vi "Dashboard Main.vi"() -> ()   [LabVIEW 2019]
uses:
  <vilib>/Utility/miscctls.llb/LVRowAndColumnTypeDef.ctl
  <vilib>/event_ctls.llb/eventvkey.ctl
  <vilib>/Rock Robotics/Network Tables/NT Write Boolean.vi
  <vilib>/Rock Robotics/WPI/Dashboard/WPI_DashboardLogging Global.vi
  <vilib>/Utility/file.llb/Write Delimited Spreadsheet (string).vi
panel:
  in  "Camera Settings Right":T1={"Frame Rate"=30, "Compression"=30, "Size"=1, "DB Camera Config"=FALSE} {"Frame Rate" scale=1.0..30.0; "Compression" scale=100.0..-1.0; "Size" items=["640x480", "320x240", "160x120"]}
  in  "Camera Name Right":string(combo)="No Camera Selection"
  out "Camera Perf":string
  in  "Camera Settings":T1={"Frame Rate"=30, "Compression"=30, "Size"=1, "DB Camera Config"=FALSE} {"Frame Rate" scale=1.0..30.0; "Compression" scale=100.0..-1.0; "Size" items=["640x480", "320x240", "160x120"]}
  in  "TCP":refnum<k5>
  in  "Rec Mode":enum32{"Stop", "Record", "Playback"}(radio)
  out "Robot IP":string
  out "Image Message":string="Timeout in Camera Communications"
  in  "Dashboard Tab":T2(tab)
  in  "Select Auto":string(combo)="Select Autonomous ..."
  out "NT Connection":bool
  out "JS1 Z":dbl(slide) scale=-1.0..1.0 scale format="%#_2e"
  out "JS1 Graph":cluster{"X":dbl, "Y":dbl}[](graph)
  out "JS1 Buttons":T3
  out "JS2 Z":dbl(slide) scale=-1.0..1.0 scale format="%#_2e"
  out "JS2 Graph":cluster{"X":dbl, "Y":dbl}[](graph)
  out "JS2 Buttons":T3
  out "Mode":T4(ring)=enum."Auto Disabled"
  out "Right Camera Perf":cluster{"Bandwidth (Mbps)":dbl, "FPS":dbl}
  out "Camera Image Right":T5(plugin-control)
  in  "DB/String 9":string
  in  "DB/String 8":string
  in  "DB/String 7":string
  in  "DB/String 6":string
  in  "DB/String 5":string
  in  "DB/String 4":string
  in  "DB/String 3":string
  in  "DB/String 2":string
  in  "DB/String 1":string
  in  "DB/String 0":string
  in  "DB/Slider 0":dbl(slide) scale=0.0..5.0
  in  "DB/Slider 1":dbl(slide) scale=0.0..5.0
  in  "DB/Slider 2":dbl(slide) scale=0.0..5.0
  in  "DB/Slider 3":dbl(slide) scale=0.0..5.0
  out "DB/LED 3":bool
  out "DB/LED 2":bool
  out "DB/LED 1":bool
  out "DB/LED 0":bool
  in  "DB/Button 3":bool
  in  "DB/Button 2":bool
  in  "DB/Button 1":bool
  in  "DB/Button 0":bool caption="New Name"
  in  "Test Slider":dbl(slide) scale=0.0..100.0 scale format="%#_3g"
  in  "On/Off":bool caption="Solenoid"
  in  "Test Name":u16(ring) items=["Select the test to run..."]
  in  "Test Tree":string(tree)
  in  "Motor":cluster{"Value":dbl, "Enable":bool} {"Value" scale=-1.0..1.0 scale format="%#_3g"}
  out "Progress":T6 {"Test Progress" scale=0.0..100.0}
  in  "Rev/Fwd":cluster{"Forward":bool, "Reverse":bool}
  in  "Test Ring":u16(ring) items=["Monochrome", "Color"]
  out "Cmd Status":string
  in  "Execute Command":bool
  in  "Command Params":string[][](table)
  in  "Command Selection":i32(listbox)
  in  "CheckList":i32(listbox)
  out "Tree":string(tree)
  out "Drive":enum32{"Controls", "Indicators"}(tab)
  in  "Left Low Gear P":dbl
  in  "Left Low Gear I":dbl
  in  "Left Low Gear D":dbl
  in  "Left Low Gear F":dbl
  in  "Left High Gear P":dbl
  in  "Left High Gear I":dbl
  in  "Left High Gear D":dbl
  in  "Left High Gear F":dbl
  in  "Right Low Gear P":dbl
  in  "Right Low Gear I":dbl
  in  "Right Low Gear D":dbl
  in  "Right Low Gear F":dbl
  in  "Right High Gear P":dbl
  in  "Right High Gear I":dbl
  in  "Right High Gear D":dbl
  in  "Right High Gear F":dbl
  out "Current Left High Gear F":dbl
  out "Current Left High Gear D":dbl
  out "Current Left High Gear P":dbl
  out "Current Left High Gear I":dbl
  out "Current Right High Gear F":dbl
  out "Current Right High Gear D":dbl
  out "Current Right High Gear P":dbl
  out "Current Right High Gear I":dbl
  out "Current Right Low Gear F":dbl
  out "Current Right Low Gear D":dbl
  out "Current Right Low Gear I":dbl
  out "Current Right Low Gear P":dbl
  out "Current Left Low Gear F":dbl
  out "Current Left Low Gear D":dbl
  out "Current Left Low Gear I":dbl
  out "Current Left Low Gear P":dbl
  out "Auto Targeting":enum32{"Controls", "Indicators"}(tab)
  in  "AutoTarget D":dbl
  in  "AutoTarget I":dbl
  in  "AutoTarget P":dbl
  out "Current AutoTarget D":dbl
  out "Current AutoTarget I":dbl
  out "Current AutoTarget P":dbl
  out "Cardinal Points":enum32{"Controls", "Indicators"}(tab)
  in  "Turret West":dbl
  in  "Turret South":dbl
  in  "Turret Safety":dbl
  in  "Turret North":dbl
  in  "Turret East":dbl
  out "Current Turret Safety":dbl
  out "Current Turret West":dbl
  out "Current Turret South":dbl
  out "Current Turret East":dbl
  out "Current Turret North":dbl
  out "Climb":enum32{"Controls", "Indicators"}(tab)
  in  "Climb I":dbl
  in  "Climb P":dbl
  in  "Climb D":dbl
  out "Current Climb D":dbl
  out "Current Climb I":dbl
  out "Current Climb P":dbl
  out "Intake":enum32{"Controls", "Indicators"}(tab)
  in  "Intake Speed":dbl
  in  "Magazine Speed":dbl
  out "Current Intake Speed":dbl
  out "Current Magazine Speed":dbl
  out "Match Color":string
  in  "Auto play selection":string
  out "Camera Image":T5(plugin-control)
  out "Background":bool
  in  "Camera Name":string(combo)="No Camera Selection"
  # "HW"
  # "HW"
  # "Joysticks"
  # "Drive Motors"
  # "Front"
  # "Right"
  # "Left"
  # "Back"
  # "This tab is a great place for autonomous settings and robot-specific values.\nPlace controls and indicators inside this tab and match name to\nDashboard Variables on robot. You can also delete this comment."
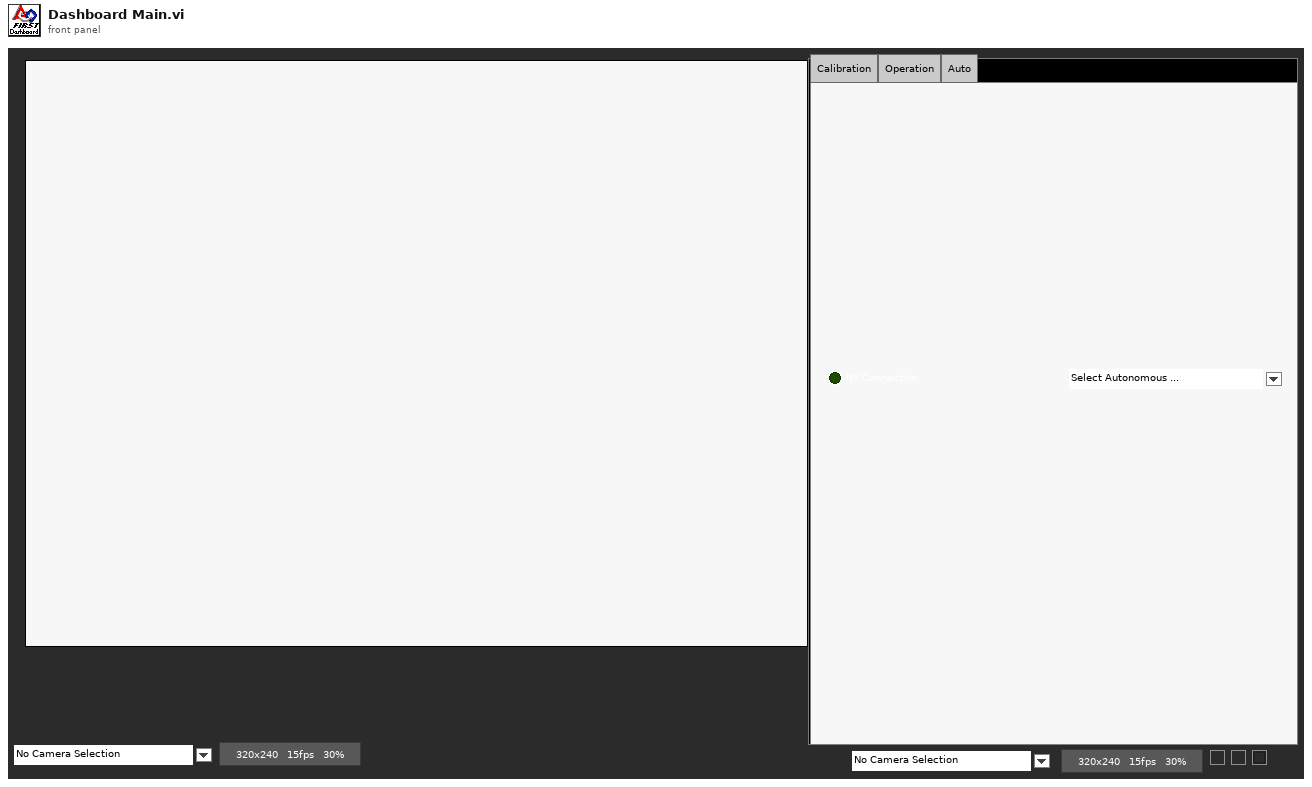
[diagram p1: front panel]
types:
  T1 = cluster{"Frame Rate":i32, "Compression":i32, "Size":u16, "DB Camera Config":bool}
  T2 = enum32{"Drive", "Camera", "Basic", "Custom", "Test", "Commands", "Checklist", "Variables", "Calibration", "Operation", "Auto"}
  T3 = cluster{bool, bool, bool, bool, bool, bool, bool, bool, bool, bool, bool, bool}
  T4 = enum8{"Tele-Op Disabled", "Tele-Op Enabled", "Auto Disabled", "Auto Enabled", "Test Disabled", "Test Enabled", "Disconnected", "No Code", "E-Stop"}
  T5 = typedef "IMAQ Image.ctl" = refnum<image>
  T6 = cluster{"Test Progress":u8, "Test Progress Text":string}
  T7 = enum16{"open", "replace", "create", "open or create", "replace or create", "replace or create with confirmation"}
  T8 = cluster{"Save Path":path, "Interval (s)":dbl, "Keep":i32}
  T9 = enum32{"Drive", "Camera", "Basic", "Custom", "Test", "Commands", "Checklist", "Variables"}
  T10 = typedef "Image Type" = u32
  T11 = cluster{"IDs":cluster{"RPC field ID":u16, "Unique ID":u16}, "String":string}
  T12 = cluster{"Error Strings":string, "Disable Counts":cluster{u16, u16}, "Rail Faults":cluster{u16, u16, u16}, "Robot IP":string, "DB Mode":u8, "Event Info":cluster{"Name":string, "Type":u8, "Number":u16, "Replay":u8}}
  T13 = cluster{"Storage":cluster{"Disk Free":u64, "RAM Block":u32, "RAM free":u32}, "CPU Utilization":cluster{"CPU % ISR":sgl, "CPU % Time Crit":sgl, "CPU % Timed Str":sgl, "CPU % High":sgl, "CPU % Above":sgl, "CPU % Normal":sgl, "CPU % Low":sgl}, "CAN":cluster{"% Bus Utilization":sgl, "Bus Off Cnt":u32, "TX_FIFO Full Cnt":u32, "Receive Error Cnt":u8, "Transmit Error Cnt":u8}, "HID":cluster{"HID Outputs":u32, "Rumble Low":u16, "Rumble High":u16}[]}
  T14 = cluster{"Status bits":cluster{"Test Mode":bool, "Autonomous":bool, "Enabled":bool, "Code Start":bool, "Brownout":bool, "Reserved 2":bool, "Reserved 3":bool, "E-Stop":bool}, "Code Trace":cluster{"Disabled":bool, "TeleOp":bool, "Auto":bool, "Test":bool}, "Controller Type":enum16{"unknown", "cRIO", "roboRio"}, "Code?":enum16{"unknown", "noCode", "code"}, "Battery V":dbl}
  T15 = cluster{"Control Bits":cluster{"TestMode":bool, "Autonomous":bool, "Enabled":bool, "FMS Present":bool, bool, bool, bool, "E-Stop":bool}, "Team Station ":u8, "Countdown":sgl, "Joystick Values":cluster{"Axes":dbl[], "Buttons":bool[], "POVs":i16[]}[]}
  T16 = cluster{"Axes":dbl[], "Buttons":bool[], "POVs":i16[]}[]
  T17 = cluster{"Axes":dbl[], "Buttons":bool[], "POVs":i16[]}
  T18 = cluster{"Buttons[0]":bool, "Buttons[1]":bool, "Buttons[2]":bool, "Buttons[3]":bool, "Buttons[4]":bool, "Buttons[5]":bool, "Buttons[6]":bool, "Buttons[7]":bool, "Buttons[8]":bool, "Buttons[9]":bool, "Buttons[10]":bool, "Buttons[11]":bool}
  T19 = cluster{"Camera Image":refnum<vi>, "Dashboard Tab":refnum<vi>, "Background":refnum<vi>, "Rec Mode":refnum<vi>, "Test Slider":refnum<vi>, "On/Off ":refnum<vi>, "Test Ring":refnum<vi>, "Rev/Fwd":refnum<vi>, "Test Name":refnum<vi>, "Motor":refnum<vi>, "Progress":refnum<vi>, "CheckList":refnum<vi>, "Tree":refnum<vi>, "Test Tree":refnum<vi>, "Command Params":refnum<vi>, "Command Selection":refnum<vi>, "Execute Command":refnum<vi>, "Cmd Status":refnum<vi>, "Camera Settings":refnum<vi>, "Camera Name":refnum<vi>, "Camera Perf":refnum<vi>, "Camera Settings Right":refnum<vi>, "Camera Name Right":refnum<vi>, "Camera Image Right":refnum<vi>}
  T20 = cluster{"Global Rectangle":i32[], "Contours":cluster{"Contour Type":u32, "ROI Type":u32, "Points":i32[]}[]}
  T21 = cluster{"Camera Name":string, string, "Saved DB Images Info":cluster{"Save Path":path, "Interval (s)":dbl, "Keep":i32}}
  T22 = cluster{"Camera Name Right":string, string, "Saved DB Images Info":cluster{"Save Path":path, "Interval (s)":dbl, "Keep":i32}}
  T23 = cluster{"Operation":enum16{"Update", "Clear"}, "Color Box":u32}[]
  T24 = typedef "eventvkey.ctl" = enum16{"ASCII", "Enter", "Return", "Shift", "Ctrl", "Alt", "Cmd", "Opt", "Caps", "NumLock", "Clear", "Break", "Up", "Down", "Left", "Right", "Insert", "Delete", "Home", "End", "PageUp", "PageDown", "Escape", "Help", "Pause", "ScrollLock", "F1", "F2", "F3", "F4", "F5", "F6", "F7", "F8", "F9", "F10", "F11", "F12", "F13", "F14", "F15", "F16", "F17", "F18", "F19", "F20", "F21", "F22", "F23", "F24", "Play", "VolumeUp", "VolumeDown", "Mute", "Two Byte Char"}
  T25 = cluster{"Image Size":bool, "Image Type":bool, "Pixel Value":bool, "ROI Information":bool, "Zoom Factor":bool}
  T26 = cluster{"Operation":enum16{"Update", "Clear"}, "Color Box":u32}
  T27 = typedef "LVRowAndColumnTypeDef.ctl" = cluster{"Row":i32, "Column":i32}
  T28 = cluster{"Shift":bool, "Ctrl":bool, "Alt":bool, "Cmd":bool, "Opt":bool}
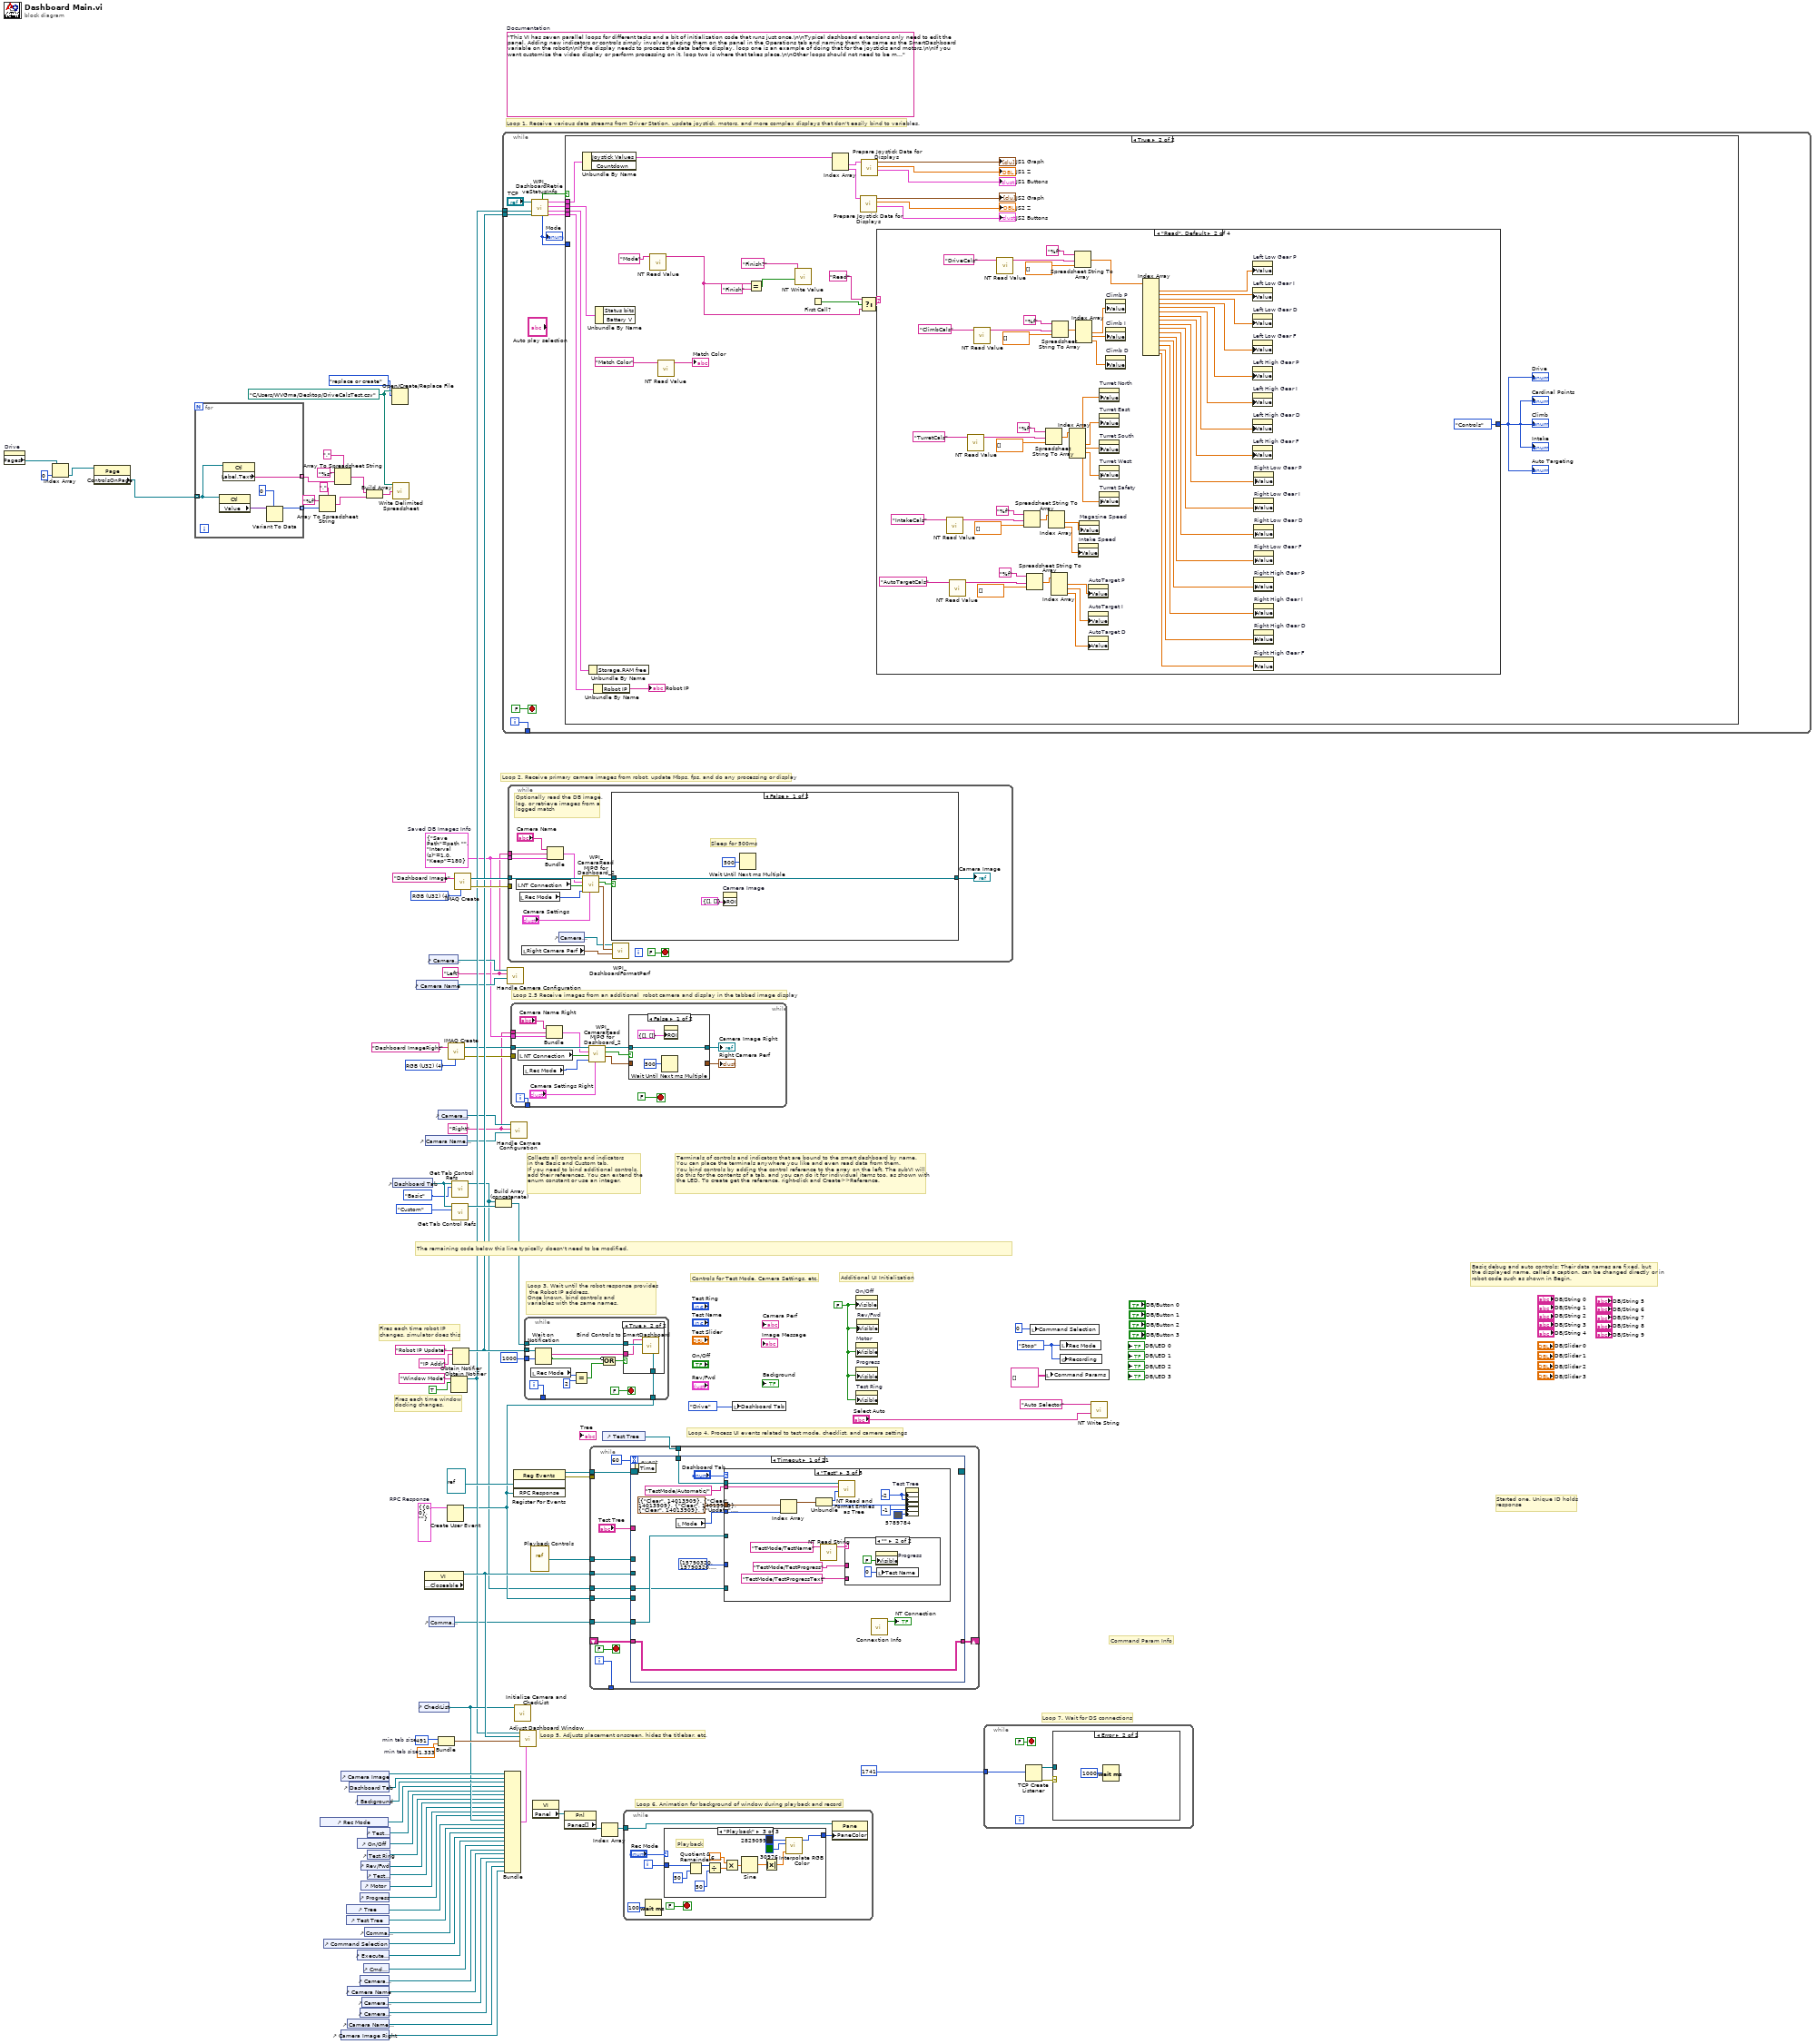
[diagram p0: block diagram]
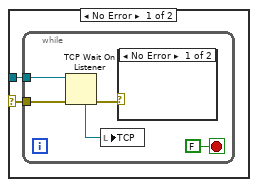
[diagram p3: hidden frame]
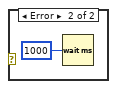
[diagram p4: hidden frame]
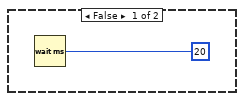
[diagram p5: hidden frame]
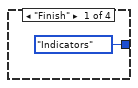
[diagram p6: hidden frame]
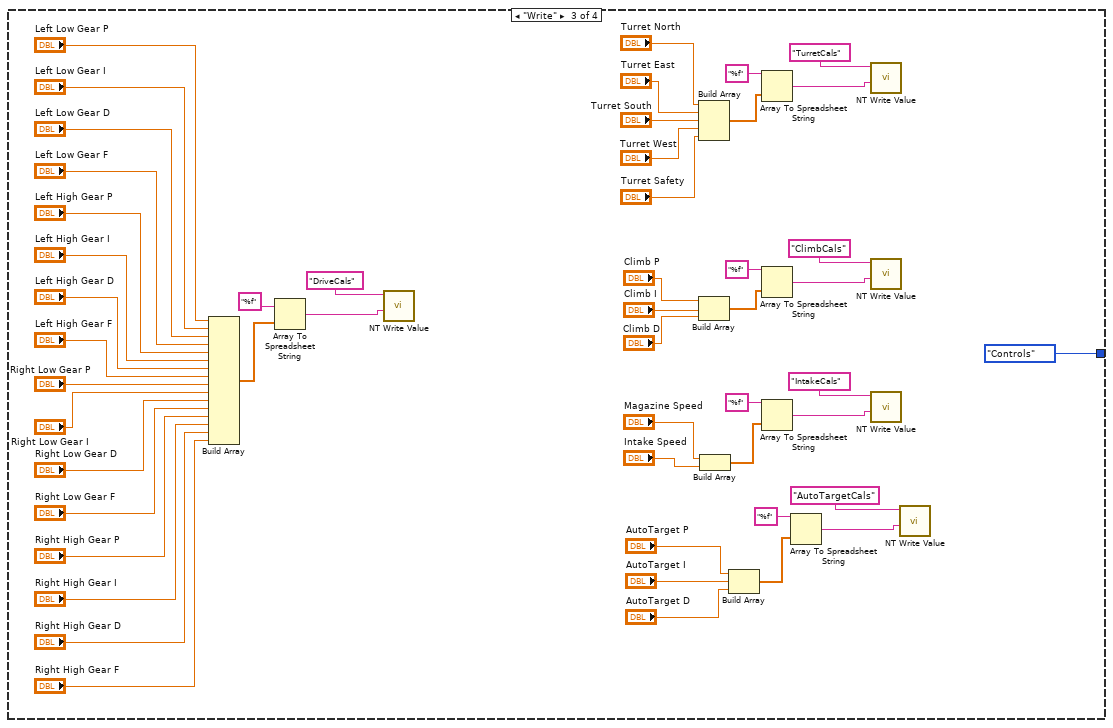
[diagram p7: hidden frame]
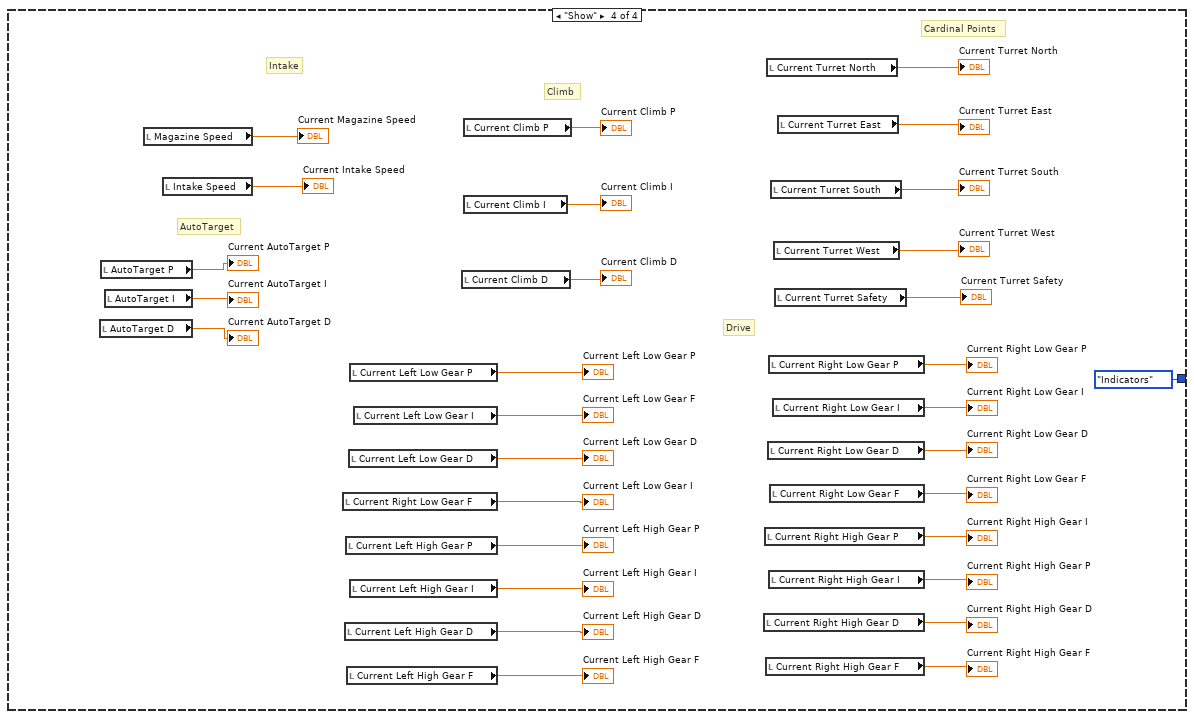
[diagram p8: hidden frame]
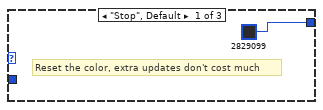
[diagram p9: hidden frame]
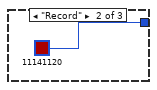
[diagram p10: hidden frame]
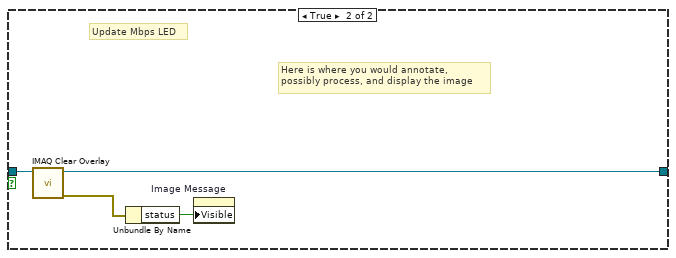
[diagram p12: hidden frame]
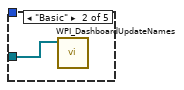
[diagram p14: hidden frame]
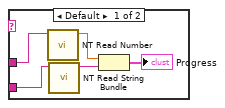
[diagram p15: hidden frame]
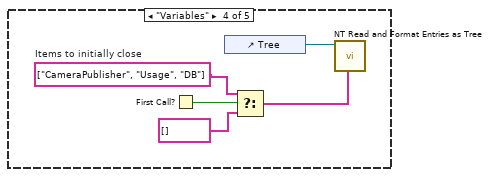
[diagram p16: hidden frame]
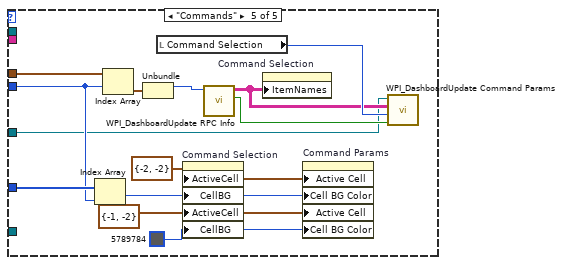
[diagram p17: hidden frame]
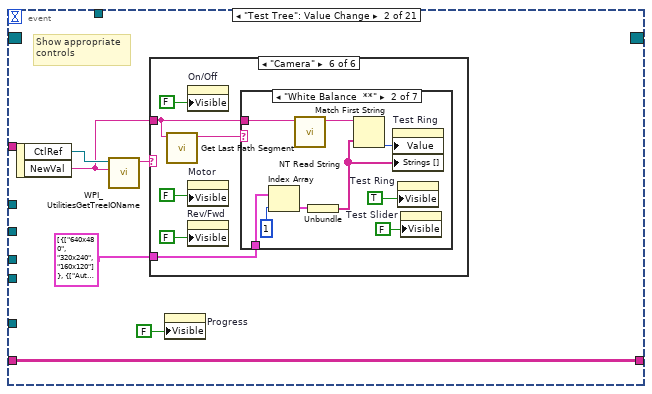
[diagram p18: hidden frame]
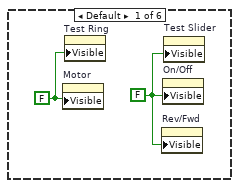
[diagram p19: hidden frame]
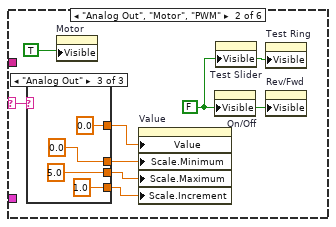
[diagram p20: hidden frame]
diagram:
  w2 = path "C:/Users/WVGma/Desktop/DriveCalsTest.csv" ("file path (dialog if empty)")
  w18 = T8 {"Save Path"=path "", "Interval (s)"=1.0, "Keep"=180}  # Saved DB Images Info
  w17 = "Right"
  w16 = "Left"
  w28 = T10 4 items=["Grayscale (U8)", "Grayscale (I16)", "Grayscale (SGL)", "Complex (CSG)", "RGB (U32)", "HSL (U32)", "RGB (U64)"] ("Image Type")
  w44 = T11 {"IDs"={"RPC field ID"=0, "Unique ID"=0}, "String"=""}  # RPC Response
  w67 = 491  # min tab size
  w66 = 1.333  # min tab size
  w74 = enum32{"Stop", "Record", "Playback"}."Stop" ("Rec Mode")
  w51 = FALSE ("Visible")
  (unwired) "This VI has seven parallel loops for different tasks and a bit of initialization code that runs just once.\n\nTypical dashboard extensions only need to edit the panel. Adding new indicators or controls simply involves placing them on the panel in the Operations tab and naming them the same as the SmartDashboard variable on the robot\n\nIf the display needs to process the data before display, loop one is an example of doing that for the joysticks and motors.\n\nIf you want customize the video display or perform processing on it, loop two is where that takes place.\n\nOther loops should not need to be modified. They are pretty standard, and document the task they perform."  # Documentation
  w91 = T10 4 items=["Grayscale (U8)", "Grayscale (I16)", "Grayscale (SGL)", "Complex (CSG)", "RGB (U32)", "HSL (U32)", "RGB (U64)"] ("Image Type")
  # "Loop 2.5 Receive images from an additional  robot camera and display in the tabbed image display"
  # "Command Param Info"
  # "Started one, Unique ID holds\nresponse"
  # "Loop 7. Wait for DS connections"
  # "Basic debug and auto controls: Their data names are fixed, but\nthe displayed name, called a caption, can be changed directly or in\nrobot code such as shown in Begin."
  # "Controls for Test Mode, Camera Settings, etc."
  # "Additional UI Initialization"
  # "Loop 6. Animation for background of window during playback and record"
  # "Fires each time robot IP\nchanges, simulator does this"
  # "Fires each time window\ndocking changes."
  # "Collects all controls and indicators\nin the Basic and Custom tab.\nIf you need to bind additional controls,\nadd their references. You can extend the\nenum constant or use an integer."
  # "The remaining code below this line typically doesn't need to be modified."
  # "Loop 4. Process UI events related to test mode, checklist, and camera settings"
  # "Terminals of controls and indicators that are bound to the smart dashboard by name.\nYou can place the terminals anywhere you like and even read data from them.\nYou bind controls by adding the control reference to the array on the left. The subVI will\ndo this for the contents of a tab, and you can do it for individual items too, as shown with\nthe LED. To create get the reference, right-click and Create>>Reference."
  # "Loop 3. Wait until the robot response provides\n the Robot IP address.\nOnce known, bind controls and\nvariables with the same names."
  # "Loop 5. Adjusts placement onscreen, hides the titlebar, etc."
  # "Loop 1. Receive various data streams from Driver Station, update joystick, motors, and more complex displays that don't easily bind to variables."
  # "Loop 2. Receive primary camera images from robot, update Mbps, fps, and do any processing or display"
  n1 = property on="Drive" class="TabCtl (strict)"() -> ("Pages"=w13:refnum<vi>[])  [unwired: 2 in, 2 out]
  n2 = Index Array(array=w13, index=0) -> (element=w14:refnum<vi>)
  n3 = property class="Page"(reference=w14) -> ("ControlsOnPage"=w15:refnum<vi>[])  [unwired: 1 in, 2 out]
  n4 = for {
    tunnel: w15 -> [w95] mode=indexing
    tunnel: [w96] -> w11 mode=indexing
    tunnel: [w92] -> w8 mode=indexing
    n5 = property class="Ctl"(reference=w95) -> ("Value"=w94:variant)  [unwired: 1 in, 2 out]
    n6 = property class="Ctl"(reference=w95) -> ("Label.Text"=w96:string)  [unwired: 1 in, 2 out]
    n7 = Variant To Data(type=0, Variant=w94) -> (data=w92:i32)  [unwired: 1 in, 1 out]
  }
  n8 = Array To Spreadsheet String(delimiter (Tab)=",", array=w8, 3:"%f" ("format string")) -> (spreadsheet string=w4:string)
  n9 = control-ref of="Rec Mode"() -> (w57:refnum<vi>)
  n10 = control-ref of="Command Selection"() -> (w43:refnum<vi>)
  n11 = Array To Spreadsheet String(delimiter (Tab)=",", array=w11, 3:"%s" ("format string")) -> (spreadsheet string=w5:string)
  n12 = control-ref of="Camera Image Right"() -> (w21:refnum<vi>)
  n13 = control-ref of="Camera Image"() -> (w69:refnum<vi>)
  n14 = control-ref of="Tree"() -> (w61:refnum<vi>)
  n15 = control-ref of="Test Tree"() -> (w60:refnum<vi>)
  n16 = control-ref of="Camera Name"() -> (w34:refnum<vi>)
  n17 = control-ref of="Camera Name Right"() -> (w22:refnum<vi>)
  n18 = control-ref of="Dashboard Tab"() -> (w68:refnum<vi>)
  n19 = control-ref of="Execute Command"() -> (w45:refnum<vi>)
  n20 = control-ref of="Background"() -> (w64:refnum<vi>)
  n21 = control-ref of="On/Off"() -> (w55:refnum<vi>)
  n22 = control-ref of="Progress"() -> (w52:refnum<vi>)
  n23 = control-ref of="Camera Settings"() -> (w35:refnum<vi>)
  n24 = control-ref of="Camera Settings Right"() -> (w23:refnum<vi>)
  n25 = control-ref of="Rev/Fwd"() -> (w53:refnum<vi>)
  n26 = control-ref of="Motor"() -> (w58:refnum<vi>)
  n27 = control-ref of="Camera Perf"() -> (w33:refnum<vi>)
  n28 = control-ref of="Cmd Status"() -> (w39:refnum<vi>)
  n29 = control-ref of="Command Params"() -> (w46:refnum<vi>)
  n30 = Build Array(w5, w4) -> (w3:string[])
  n31 = control-ref of="Test Slider"() -> (w56:refnum<vi>)
  n32 = control-ref of="Test Ring"() -> (w54:refnum<vi>)
  n33 = control-ref of="Test Name"() -> (w59:refnum<vi>)
  n34 = Open/Create/Replace File(file path (use dialog)=w2, operation (0:open)=T7."replace or create") -> ()  [unwired: 4 in, 3 out]
  n35 = call-poly <vilib>:"Write Delimited Spreadsheet.vi"("file path (dialog if empty)"=w2, "1D data"=w3) -> ()  [unwired: 12 in, 2 out]
  n36 = control-ref of="Dashboard Tab"() -> (w72:refnum<vi>)
  n37 = control-ref of="Camera Name"() -> (w36:refnum<vi>)
  n38 = control-ref of="CheckList"() -> (w62:refnum<vi>)
  n39 = property class="VI" props=["Front Panel.Closeable"]() -> (reference out=w73:refnum<vi>)  [unwired: 2 in, 2 out]
  n40 = control-ref of="Camera Name Right"() -> (w24:refnum<vi>)
  n41 = control-ref of="Camera Settings"() -> (w37:refnum<vi>)
  n42 = control-ref of="Command Params"() -> (w38:refnum<vi>)
  n43 = control-ref of="Camera Settings Right"() -> (w25:refnum<vi>)
  n44 = Bundle("min tab size"=w67, "min tab size"=w66) -> (w65:cluster{"min tab size":i32, "min tab size":dbl})  [unwired: 1 in]
  n45 = Create User Event(user event datatype=w44) -> (user event=w40:refnum<user-event>)  [unwired: 1 in, 1 out]
  n46 = call "IMAQ Create"("Image Name"="Dashboard ImageRight", "Image Type"=w28) -> ("New Image"=w27:T5, "error out"=w26:errorcluster)  [unwired: 2 in, 1 out]
  n47 = Obtain Notifier(name (unnamed)="Window Mode", notification data type=TRUE) -> (notifier out=w49:refnum<notifier>)  [unwired: 2 in, 2 out]
  n48 = call <vilib>:"Get Tab Control Refs.vi"("Page Index"=T9."Basic" ("Dashboard Tab"), "TabControl in"=w72) -> ("ControlsOnPage"=w32:refnum<vi>[])  [unwired: 9 in]
  n49 = call <vilib>:"Get Tab Control Refs.vi"("Page Index"=T9."Custom" ("Dashboard Tab"), "TabControl in"=w72) -> ("ControlsOnPage"=w71:refnum<vi>[])  [unwired: 9 in]
  n50 = Obtain Notifier(name (unnamed)="Robot IP Update", notification data type="IP Addr" ("name (unnamed)")) -> (notifier out=w50:refnum<notifier>)  [unwired: 2 in, 2 out]
  n51 = call "IMAQ Create"("Image Name"="Dashboard Image", "Image Type"=w91) -> ("New Image"=w89:T5, "error out"=w88:errorcluster)  [unwired: 2 in, 1 out]
  n52 = Build Array (concatenate)(w32, w71) -> (w70:refnum<vi>[])
  n53 = while {
    tunnel: [w106] -> _
    tunnel: w50 -> [w100]
    tunnel: w49 -> [w97]
    i -> [w106]
    stop <- FALSE stop-if-true
    n54 = call <vilib>:"WPI_DashboardRetrieveStatusInfo.vi"("Binding Refnum"=w100, "Window Mode Notifier"=w97, "TCP Cnx"="TCP") -> ("Power and Errors"=w101:T12, "Robot Metrics"=w104:T13, "Status Info"=w105:T14, "Control Info"=w102:T15, "Robot Mode"=w99:T4, "Process?"=w103:bool)  [unwired: 3 in]
    "Mode" <- w99
    n55 = case shown="True" w103 {
      tunnel: w105 -> [_ w133]
      tunnel: w104 -> [_ w132]
      tunnel: w102 -> [_ w131]
      tunnel: w101 -> [_ w130]
      tunnel: w99 -> [_ _]
      frame False {
        n56 = Wait (ms)(milliseconds to wait=u32 20) -> ()  [unwired: 1 out]
      }
      frame True {
        n57 = Unbundle By Name(w131) -> ("Joystick Values"=w129:T16)  [unwired: 1 out]
        n58 = Unbundle By Name(w132) -> ()  [unwired: 1 out]
        n59 = Unbundle By Name(w130) -> ("Robot IP"=→"Robot IP":string)
        n60 = Unbundle By Name(w133) -> ()  [unwired: 2 out]
        n61 = call-poly <vilib>:"NT Read Value.vi"("Name"="Mode") -> ("String"=w113:string)  [unwired: 9 in, 1 out]
        n62 = call-poly <vilib>:"NT Read Value.vi"("Name"="Match Color") -> ("String"=→"Match Color":string)  [unwired: 9 in, 1 out]
        n63 = Equal?(x=w113, y="Finish") -> (x = y?=w117:bool)
        n64 = call-poly <vilib>:"NT Write Value.vi"("Boolean"=w117, "Name"="Finish?") -> ()  [unwired: 9 in, 1 out]
        n65 = First Call?() -> (First Call?: T/F=w115:bool)
        n66 = Index Array(array=w129) -> (element #1=w128:T17, element #2=w124:T17)  [unwired: 2 in]
        n67 = call "Prepare Joystick Data for Displays.vi"("Joystick Values"=w124) -> ("Buttons"=→"JS2 Buttons":T18, "Z Axis"=→"JS2 Z":dbl, "Cartesian Data"=→"JS2 Graph":cluster{"X axis":dbl, "X axis":dbl}[])  [unwired: 8 in]
        n68 = call "Prepare Joystick Data for Displays.vi"("Joystick Values"=w128) -> ("Buttons"=→"JS1 Buttons":T18, "Z Axis"=→"JS1 Z":dbl, "Cartesian Data"=→"JS1 Graph":cluster{"X axis":dbl, "X axis":dbl}[])  [unwired: 8 in]
        n69 = Select(t="Read" ("f"), s=w115, f=w113) -> (s? t:f=w112:string)
        n70 = case shown="\"Read\", Default" w112 {
          tunnel: [enum32{"Controls", "Indicators"}."Indicators" ("Climb") enum32{"Controls", "Indicators"}."Controls" ("Climb") enum32{"Controls", "Indicators"}."Controls" ("Climb") enum32{"Controls", "Indicators"}."Indicators" ("Climb")] -> w109
          frame "Finish" {
          }
          frame "Read", Default {
            n71 = call-poly <vilib>:"NT Read Value.vi"("Name"="IntakeCals") -> ("String"=w146:string)  [unwired: 9 in, 1 out]
            n72 = call-poly <vilib>:"NT Read Value.vi"("Name"="AutoTargetCals") -> ("String"=w139:string)  [unwired: 9 in, 1 out]
            n73 = call-poly <vilib>:"NT Read Value.vi"("Name"="TurretCals") -> ("String"=w156:string)  [unwired: 9 in, 1 out]
            n74 = call-poly <vilib>:"NT Read Value.vi"("Name"="ClimbCals") -> ("String"=w163:string)  [unwired: 9 in, 1 out]
            n75 = call-poly <vilib>:"NT Read Value.vi"("Name"="DriveCals") -> ("String"=w185:string)  [unwired: 9 in, 1 out]
            n76 = Spreadsheet String To Array(format string="%f", spreadsheet string=w146, array type (2D Dbl)=dbl[] []) -> (array=w145:dbl[])  [unwired: 1 in]
            n77 = Spreadsheet String To Array(format string="%f", spreadsheet string=w139, array type (2D Dbl)=dbl[] []) -> (array=w138:dbl[])  [unwired: 1 in]
            n78 = Spreadsheet String To Array(format string="%f", spreadsheet string=w156, array type (2D Dbl)=dbl[] []) -> (array=w155:dbl[])  [unwired: 1 in]
            n79 = Index Array(array=w145) -> (element #1=w144:dbl, element #2=w143:dbl)  [unwired: 2 in]
            n80 = Index Array(array=w138) -> (element #1=w137:dbl, element #2=w136:dbl, element #3=w135:dbl)  [unwired: 3 in]
            n81 = Spreadsheet String To Array(format string="%f", spreadsheet string=w163, array type (2D Dbl)=dbl[] []) -> (array=w166:dbl[])  [unwired: 1 in]
            n82 = Index Array(array=w155) -> (element #1=w152:dbl, element #2=w153:dbl, element #3=w154:dbl, element #4=w151:dbl, element #5=w150:dbl)  [unwired: 5 in]
            n83 = Spreadsheet String To Array(format string="%f", spreadsheet string=w185, array type (2D Dbl)=dbl[] []) -> (array=w188:dbl[])  [unwired: 1 in]
            n84 = Index Array(array=w166) -> (element #1=w162:dbl, element #2=w161:dbl, element #3=w160:dbl)  [unwired: 3 in]
            n85 = property on="Intake Speed" class="DigNum (strict)"("Value"=w143) -> ()  [unwired: 2 in, 2 out]
            n86 = property on="Magazine Speed" class="DigNum (strict)"("Value"=w144) -> ()  [unwired: 2 in, 2 out]
            n87 = property on="AutoTarget P" class="DigNum (strict)"("Value"=w137) -> ()  [unwired: 2 in, 2 out]
            n88 = property on="AutoTarget I" class="DigNum (strict)"("Value"=w136) -> ()  [unwired: 2 in, 2 out]
            n89 = property on="AutoTarget D" class="DigNum (strict)"("Value"=w135) -> ()  [unwired: 2 in, 2 out]
            n90 = property on="Turret North" class="DigNum (strict)"("Value"=w152) -> ()  [unwired: 2 in, 2 out]
            n91 = property on="Turret East" class="DigNum (strict)"("Value"=w153) -> ()  [unwired: 2 in, 2 out]
            n92 = property on="Turret South" class="DigNum (strict)"("Value"=w154) -> ()  [unwired: 2 in, 2 out]
            n93 = property on="Turret West" class="DigNum (strict)"("Value"=w151) -> ()  [unwired: 2 in, 2 out]
            n94 = property on="Turret Safety" class="DigNum (strict)"("Value"=w150) -> ()  [unwired: 2 in, 2 out]
            n95 = property on="Climb P" class="DigNum (strict)"("Value"=w162) -> ()  [unwired: 2 in, 2 out]
            n96 = property on="Climb I" class="DigNum (strict)"("Value"=w161) -> ()  [unwired: 2 in, 2 out]
            n97 = property on="Climb D" class="DigNum (strict)"("Value"=w160) -> ()  [unwired: 2 in, 2 out]
            n98 = Index Array(array=w188) -> (element #1=w168:dbl, element #2=w169:dbl, element #3=w170:dbl, element #4=w171:dbl, element #5=w172:dbl, element #6=w173:dbl, element #7=w174:dbl, element #8=w175:dbl, element #9=w176:dbl, element #10=w177:dbl, element #11=w178:dbl, element #12=w179:dbl, element #13=w180:dbl, element #14=w181:dbl, element #15=w182:dbl, element #16=w183:dbl)  [unwired: 16 in]
            n99 = property on="Left Low Gear P" class="DigNum (strict)"("Value"=w168) -> ()  [unwired: 2 in, 2 out]
            n100 = property on="Left Low Gear I" class="DigNum (strict)"("Value"=w169) -> ()  [unwired: 2 in, 2 out]
            n101 = property on="Left Low Gear D" class="DigNum (strict)"("Value"=w170) -> ()  [unwired: 2 in, 2 out]
            n102 = property on="Left Low Gear F" class="DigNum (strict)"("Value"=w171) -> ()  [unwired: 2 in, 2 out]
            n103 = property on="Left High Gear P" class="DigNum (strict)"("Value"=w172) -> ()  [unwired: 2 in, 2 out]
            n104 = property on="Left High Gear I" class="DigNum (strict)"("Value"=w173) -> ()  [unwired: 2 in, 2 out]
            n105 = property on="Left High Gear D" class="DigNum (strict)"("Value"=w174) -> ()  [unwired: 2 in, 2 out]
            n106 = property on="Left High Gear F" class="DigNum (strict)"("Value"=w175) -> ()  [unwired: 2 in, 2 out]
            n107 = property on="Right Low Gear P" class="DigNum (strict)"("Value"=w176) -> ()  [unwired: 2 in, 2 out]
            n108 = property on="Right Low Gear I" class="DigNum (strict)"("Value"=w177) -> ()  [unwired: 2 in, 2 out]
            n109 = property on="Right Low Gear D" class="DigNum (strict)"("Value"=w178) -> ()  [unwired: 2 in, 2 out]
            n110 = property on="Right Low Gear F" class="DigNum (strict)"("Value"=w179) -> ()  [unwired: 2 in, 2 out]
            n111 = property on="Right High Gear P" class="DigNum (strict)"("Value"=w180) -> ()  [unwired: 2 in, 2 out]
            n112 = property on="Right High Gear I" class="DigNum (strict)"("Value"=w181) -> ()  [unwired: 2 in, 2 out]
            n113 = property on="Right High Gear D" class="DigNum (strict)"("Value"=w182) -> ()  [unwired: 2 in, 2 out]
            n114 = property on="Right High Gear F" class="DigNum (strict)"("Value"=w183) -> ()  [unwired: 2 in, 2 out]
          }
          frame "Write" {
            n115 = Build Array("Left Low Gear P", "Left Low Gear I", "Left Low Gear D", "Left Low Gear F", "Left High Gear P", "Left High Gear I", "Left High Gear D", "Left High Gear F", "Right Low Gear P", "Right Low Gear I", "Right Low Gear D", "Right Low Gear F", "Right High Gear P", "Right High Gear I", "Right High Gear D", "Right High Gear F") -> (w237:dbl[])
            n116 = Array To Spreadsheet String(array=w237, 3:"%f" ("format string")) -> (spreadsheet string=w238:string)  [unwired: 1 in]
            n117 = call-poly <vilib>:"NT Write Value.vi"("String"=w238, "Name"="DriveCals") -> ()  [unwired: 9 in, 1 out]
            n118 = Build Array("Turret North", "Turret East", "Turret South", "Turret West", "Turret Safety") -> (w217:dbl[])
            n119 = Build Array("Climb P", "Climb I", "Climb D") -> (w208:dbl[])
            n120 = Build Array("Magazine Speed", "Intake Speed") -> (w200:dbl[])
            n121 = Build Array("AutoTarget P", "AutoTarget I", "AutoTarget D") -> (w194:dbl[])
            n122 = Array To Spreadsheet String(array=w217, 3:"%f" ("format string")) -> (spreadsheet string=w219:string)  [unwired: 1 in]
            n123 = Array To Spreadsheet String(array=w208, 3:"%f" ("format string")) -> (spreadsheet string=w210:string)  [unwired: 1 in]
            n124 = Array To Spreadsheet String(array=w200, 3:"%f" ("format string")) -> (spreadsheet string=w203:string)  [unwired: 1 in]
            n125 = Array To Spreadsheet String(array=w194, 3:"%f" ("format string")) -> (spreadsheet string=w197:string)  [unwired: 1 in]
            n126 = call-poly <vilib>:"NT Write Value.vi"("String"=w219, "Name"="TurretCals") -> ()  [unwired: 9 in, 1 out]
            n127 = call-poly <vilib>:"NT Write Value.vi"("String"=w210, "Name"="ClimbCals") -> ()  [unwired: 9 in, 1 out]
            n128 = call-poly <vilib>:"NT Write Value.vi"("String"=w203, "Name"="IntakeCals") -> ()  [unwired: 9 in, 1 out]
            n129 = call-poly <vilib>:"NT Write Value.vi"("String"=w197, "Name"="AutoTargetCals") -> ()  [unwired: 9 in, 1 out]
          }
          frame "Show" {
            # "AutoTarget"
            # "Intake"
            # "Climb"
            # "Cardinal Points"
            # "Drive"
            n130 = local read "AutoTarget D"() -> (→"Current AutoTarget D":dbl)
            n131 = local read "AutoTarget P"() -> (→"Current AutoTarget P":dbl)
            n132 = local read "AutoTarget I"() -> (→"Current AutoTarget I":dbl)
            n133 = local read "Magazine Speed"() -> (→"Current Magazine Speed":dbl)
            n134 = local read "Intake Speed"() -> (→"Current Intake Speed":dbl)
            n135 = local read "Current Right Low Gear F"() -> (→"Current Left Low Gear I":dbl)
            n136 = local read "Current Left High Gear D"() -> (→"Current Left High Gear D":dbl)
            n137 = local read "Current Left High Gear P"() -> (→"Current Left High Gear P":dbl)
            n138 = local read "Current Left High Gear F"() -> (→"Current Left High Gear F":dbl)
            n139 = local read "Current Left Low Gear D"() -> (→"Current Left Low Gear D":dbl)
            n140 = local read "Current Left Low Gear P"() -> (→"Current Left Low Gear P":dbl)
            n141 = local read "Current Left High Gear I"() -> (→"Current Left High Gear I":dbl)
            n142 = local read "Current Left Low Gear I"() -> (→"Current Left Low Gear F":dbl)
            n143 = local read "Current Climb D"() -> (→"Current Climb D":dbl)
            n144 = local read "Current Climb P"() -> (→"Current Climb P":dbl)
            n145 = local read "Current Climb I"() -> (→"Current Climb I":dbl)
            n146 = local read "Current Right High Gear D"() -> (→"Current Right High Gear D":dbl)
            n147 = local read "Current Right High Gear P"() -> (→"Current Right High Gear I":dbl)
            n148 = local read "Current Right High Gear F"() -> (→"Current Right High Gear F":dbl)
            n149 = local read "Current Turret North"() -> (→"Current Turret North":dbl)
            n150 = local read "Current Right Low Gear D"() -> (→"Current Right Low Gear D":dbl)
            n151 = local read "Current Right Low Gear P"() -> (→"Current Right Low Gear P":dbl)
            n152 = local read "Current Right High Gear I"() -> (→"Current Right High Gear P":dbl)
            n153 = local read "Current Right Low Gear F"() -> (→"Current Right Low Gear F":dbl)
            n154 = local read "Current Turret South"() -> (→"Current Turret South":dbl)
            n155 = local read "Current Right Low Gear I"() -> (→"Current Right Low Gear I":dbl)
            n156 = local read "Current Turret West"() -> (→"Current Turret West":dbl)
            n157 = local read "Current Turret Safety"() -> (→"Current Turret Safety":dbl)
            n158 = local read "Current Turret East"() -> (→"Current Turret East":dbl)
          }
        }
        "Drive" <- w109
        "Cardinal Points" <- w109
        "Climb" <- w109
        "Auto Targeting" <- w109
        "Intake" <- w109
      }
    }
  }
  n159 = Bundle("Camera Image"=w69, "Dashboard Tab"=w68, "Background"=w64, "Rec Mode"=w57, "Test Slider"=w56, "On/Off"=w55, "Test Ring"=w54, "Rev/Fwd"=w53, "Test Name"=w59, "Motor"=w58, "Progress"=w52, "CheckList"=w62, "Tree"=w61, "Test Tree"=w60, "Command Params"=w46, "Command Selection"=w43, "Execute Command"=w45, "Cmd Status"=w39, "Camera Settings"=w35, "Camera Name"=w34, "Camera Perf"=w33, "Camera Settings Right"=w23, "Camera Name Right"=w22, "Camera Image Right"=w21) -> (w63:T19)  [unwired: 1 in]
  n160 = call "Handle Camera Configuration.vi"("CameraNameRef"=w36, "Display Name"=w16, "ClusterRef"=w37) -> ()  [unwired: 9 in]
  n161 = while {
    tunnel: w89 -> [w283]
    tunnel: w88 -> [_]
    tunnel: w18 -> [w276]
    tunnel: w16 -> [w273]
    stop <- FALSE stop-if-true
    # "Optionally read the DB image,\nlog, or retrieve images from a\nlogged match"
    n162 = local read "NT Connection"() -> (w277:bool)
    n163 = local read "Rec Mode"() -> (w280:enum32{"Stop", "Record", "Playback"})
    n164 = local read "Right Camera Perf"() -> (w271:cluster{"Bandwidth (Mbps)":dbl, "FPS":dbl})
    n165 = Bundle("Camera Name"="Camera Name", w273, "Saved DB Images Info"=w276) -> (w275:T21)  [unwired: 1 in]
    n166 = control-ref of="Camera Perf"() -> (w270:refnum<vi>)
    n167 = call <vilib>:"WPI_CameraRead MJPG for Dashboard_2.vi"("Camera Settings"="Camera Settings", "Rec Mode"=w280, "NT Connection"=w277, "Capture Info"=w275, "Image in"=w283) -> ("perf info"=w272:cluster{"Bandwidth (Mbps)":dbl, "fps":dbl}, "Active"=w281:bool, "Image\\ out"=w282:T5)  [unwired: 4 in]
    n168 = case shown="False" w281 {
      tunnel: w282 -> [w286 w289]
      tunnel: [w286 w288] -> w278
      frame False {
        # "Sleep for 500ms"
        n169 = property on="Camera Image" class="ImageControl"("ROI"=T20 {"Global Rectangle"=[], "Contours"=[]}) -> ()  [unwired: 2 in, 2 out]
        n170 = Wait Until Next ms Multiple(millisecond multiple=u32 500) -> ()  [unwired: 1 out]
      }
      frame True {
        # "Here is where you would annotate,\npossibly process, and display the image"
        # "Update Mbps LED"
        n171 = call "IMAQ Clear Overlay"("Image"=w289) -> ("error out"=w290:errorcluster, "Image Out"=w288:T5)  [unwired: 2 in, 7 out]
        n172 = Unbundle By Name(w290) -> ("status"=w291:bool)
        n173 = property on="Image Message" class="Str"("Visible"=w291) -> ()  [unwired: 2 in, 2 out]
      }
    }
    "Camera Image" <- w278
    n174 = call <vilib>:"WPI_DashboardFormatPerf.vi"("Right Camera Perf"=w271, "Performance"=w272, "String in"=w270) -> ()  [unwired: 9 in]
  }
  n175 = call "Handle Camera Configuration.vi"("CameraNameRef"=w24, "Display Name"=w17, "ClusterRef"=w25) -> ()  [unwired: 9 in]
  n176 = while {
    tunnel: w27 -> [w306]
    tunnel: w26 -> [_]
    tunnel: [w301] -> _
    tunnel: w18 -> [w297]
    tunnel: w17 -> [w294]
    i -> [w301]
    stop <- FALSE stop-if-true
    n177 = local read "NT Connection"() -> (w298:bool)
    n178 = local read "Rec Mode"() -> (w305:enum32{"Stop", "Record", "Playback"})
    n179 = Bundle("Camera Name Right"="Camera Name Right", w294, "Saved DB Images Info"=w297) -> (w296:T22)  [unwired: 1 in]
    n180 = call <vilib>:"WPI_CameraRead MJPG for Dashboard_2.vi"("Camera Settings"="Camera Settings Right", "Rec Mode"=w305, "NT Connection"=w298, "Capture Info"=w296, "Image in"=w306) -> ("perf info"=w292:cluster{"Bandwidth (Mbps)":dbl, "fps":dbl}, "Active"=w300:bool, "Image\\ out"=w303:T5)  [unwired: 4 in]
    n181 = case shown="False" w300 {
      tunnel: w303 -> [w308 w311]
      tunnel: [w308 w311] -> w299
      tunnel: [_ w310] -> w293
      tunnel: w292 -> [_ w310]
      frame False {
        n182 = Wait Until Next ms Multiple(millisecond multiple=u32 500) -> ()  [unwired: 1 out]
        n183 = property on="Camera Image Right" class="ImageControl"("ROI"=T20 {"Global Rectangle"=[], "Contours"=[]}) -> ()  [unwired: 2 in, 2 out]
      }
      frame True {
      }
    }
    "Camera Image Right" <- w299
    "Right Camera Perf" <- w293
  }
  n184 = register-events(refnum<vi> refnum, w40) -> (reference out=w78:refnum<event-registration>, error out=w77:errorcluster)  [unwired: 2 in]
  n185 = call "Initialize Camera and CheckList.vi"("ListBox in"=w62) -> ()  [unwired: 11 in]
  n186 = call "Adjust Dashboard Window.vi"("Sizing Refnums"=w63, "Size Constraints"=w65, "VI"=w73, "WIn Mode"=w49) -> ()  [unwired: 8 in]
  n187 = while {
    tunnel: w70 -> [w323]
    tunnel: w50 -> [w321]
    tunnel: [w319] -> _
    tunnel: u32 1000 ("milliseconds to wait") -> [w318]
    tunnel: w40 -> [w312]
    i -> [w319]
    stop <- FALSE stop-if-true
    n188 = local read "Rec Mode"() -> (w314:enum32{"Stop", "Record", "Playback"})
    n189 = Wait on Notification(notifier=w321, timeout in ms (-1)=w318) -> (notification=w320:string, timed out?=w316:bool)  [unwired: 2 in, 2 out]
    n190 = Equal?(x=w314, y=u16 2 ("Rec Mode")) -> (x = y?=w315:bool)
    n191 = Compound Arithmetic op=OR(invert w316, w315) -> (w317:bool)
    n192 = case shown="True" w317 {
      tunnel: w323 -> [_ w326]
      tunnel: w320 -> [_ w325]
      tunnel: w312 -> [_ w324]
      frame False {
      }
      frame True {
        n193 = call <vilib>:"Bind Controls to SmartDashboard.vi"("RPC ref"=w324, "Bound Control Refs"=w326, "Server IP Address"=w325) -> ()  [unwired: 9 in]
      }
    }
  }
  n194 = vi-ref "Playback Controls.vi"() -> (w79:refnum<vi>)
  n195 = property class="VI"() -> ("Panel"=w81:refnum<vi>)  [unwired: 2 in, 2 out]
  n196 = property class="Pnl"(reference=w81) -> ("Panes[]"=w82:refnum<vi>[])  [unwired: 1 in, 2 out]
  n197 = Index Array(array=w82) -> (element=w80:refnum<vi>)  [unwired: 1 in]
  n198 = control-ref of="Test Tree"() -> (w83:refnum<vi>)
  n199 = while {
    tunnel: [w336] -> _
    tunnel: w83 -> [w335]
    tunnel: w79 -> [w334]
    tunnel: w78 -> [w333]
    tunnel: w77 -> [_]
    tunnel: w73 -> [w332]
    tunnel: w40 -> [w331]
    tunnel: w38 -> [w330]
    shift-right: [w329] -> _
    shift-left: _ -> [w328]
    tunnel: w32 -> [w327]
    i -> [w336]
    stop <- FALSE stop-if-true
    n200 = event shown="[0] Timeout" {
      selector: w333 -> [_ _ _ _ _ _ _ _ _ _ _ _ _ _ _ _ _ _ _ _ _]
      dyn-events: [_ _ _ _ _ _ _ _ _ _ _ _ _ _ _ _ w596 _ _ _ _] -> _
      timeout: u32 60 ("milliseconds to wait") -> [_ _ _ _ _ _ _ _ _ _ _ _ _ _ _ _ _ _ _ _ _]
      tunnel: w335 -> [w348 _ _ _ _ _ _ _ _ _ _ _ _ _ _ _ _ _ _ _ _]
      tunnel: "Test Tree" -> [_ _ _ _ _ _ _ _ _ _ _ w563 w571 w573 w577 w585 _ _ _ _ _]
      tunnel: w334 -> [_ _ _ _ _ _ _ _ _ _ _ _ _ _ _ _ w598 _ w616 _ _]
      tunnel: w332 -> [_ _ _ _ _ _ _ _ _ _ _ _ _ _ _ _ w594 _ _ _ _]
      tunnel: w331 -> [_ _ _ _ _ _ _ _ _ _ _ _ _ _ _ _ w592 _ _ _ _]
      tunnel: w330 -> [w343 _ _ _ _ _ w514 _ _ _ _ _ _ _ _ _ _ _ _ _ _]
      tunnel: [w342 w391 w493 w498 w507 w511 w512 w521 w531 w538 w550 w562 w569 w572 w576 w584 w591 w611 w613 w617 w630] -> w329
      tunnel: w328 -> [w342 w391 w493 w498 w507 w511 w512 _ _ w538 w550 w562 w569 w572 w576 w584 w591 w611 w613 w617 w630]
      tunnel: w327 -> [w340 _ _ _ _ _ _ _ _ _ _ _ _ _ _ _ _ _ _ _ _]
      event Timeout {
        n201 = event-data() -> ()  [unwired: 1 in, 1 out]
        n202 = local read "Mode"() -> (w345:T4)
        n203 = case shown="\"Test\"" "Dashboard Tab" {
          tunnel: w348 -> [_ _ w364 _ _]
          tunnel: "TestMode/Automatic/" ("Name Pattern") -> [_ _ w363 _ _]
          tunnel: T23 [{"Operation"=enum."Clear", "Color Box"=14013909}, {"Operation"=enum."Clear", "Color Box"=14013909}, {"Operation"=enum."Clear", "Color Box"=14013909}, {"Operation"=enum."Clear", "Color Box"=14013909}, {"Operation"=enum."Update", "Color Box"=14013909}, {"Operation"=enum."Update", "Color Box"=16777215}, {"Operation"=enum."Clear", "Color Box"=14013909}, {"Operation"=enum."Clear", "Color Box"=14013909}, {"Operation"=enum."Clear", "Color Box"=14013909}] -> [_ _ w356 _ w384]
          tunnel: w345 -> [_ _ w355 _ w383]
          tunnel: u32[] [15790320, 15790320, 15790320, 15790320, 16777215, 16777215, 15790320, 15790320, 15790320] -> [_ _ _ _ w389]
          tunnel: w343 -> [_ _ _ _ w377]
          tunnel: w340 -> [_ w350 _ _ _]
          frame "Custom", Default {
          }
          frame "Basic" {
            n204 = call <vilib>:"WPI_DashboardUpdateNames.vi"("Controls on Tab"=w350) -> ()  [unwired: 11 in]
          }
          frame "Test" {
            w362 = -2 ("Active Item:Row Number")
            n205 = Index Array(array=w356, index=w355) -> (element=w357:T26)
            n206 = Unbundle(w357) -> ("Operation"=w358:enum16{"Update", "Clear"}, "Color Box"=w359:u32)
            n207 = call <vilib>:"NT Read String.vi"("Name"="TestMode/TestName") -> ("String"=w353:string)  [unwired: 9 in, 1 out]
            n208 = call <vilib>:"NT Read and Format Entries as Tree.vi"("Operation"=w358, "Name Pattern"=w363, "Tree Refnum"=w364) -> ()  [unwired: 7 in, 2 out]
            n209 = case shown="\"\"" w353 {
              tunnel: "TestMode/TestProgress" ("Name") -> [w366 _]
              tunnel: "TestMode/TestProgressText" ("Name") -> [w365 _]
              frame Default {
                n210 = call <vilib>:"NT Read Number.vi"("Name"=w366) -> ("Numeric"=w367:dbl)  [unwired: 9 in, 1 out]
                n211 = call <vilib>:"NT Read String.vi"("Name"=w365) -> ("String"=w368:string)  [unwired: 9 in, 1 out]
                n212 = Bundle("Numeric"=w367, "String"=w368) -> (→"Progress":cluster{"Numeric":dbl, "String":string})  [unwired: 1 in]
              }
              frame "" {
                n213 = property on="Progress" class="Clust (strict)"("Visible"=FALSE) -> ()  [unwired: 2 in, 2 out]
                n214 = local write "Test Name"(u16 0) -> ()
              }
            }
            n215 = property on="Test Tree" class="Tree (strict)"("Active Item Row Number"=w362, "ActiveColNum"=w362, "CellBG"=w359, "Active Item Row Number"=-1 ("Active Item:Row Number"), "CellBG"=u32 5789784 ("Color Box")) -> ()  [unwired: 2 in, 2 out]
          }
          frame "Variables" {
            w374 = string[] ["CameraPublisher", "Usage", "DB"]  # Items to initially close
            n216 = First Call?() -> (First Call?: T/F=w375:bool)
            n217 = control-ref of="Tree"() -> (w376:refnum<vi>)
            n218 = Select(t=w374, s=w375, f=string[] []) -> (s? t:f=w372:string[])
            n219 = call <vilib>:"NT Read and Format Entries as Tree.vi"("Tags to  Close"=w372, "Tree Refnum"=w376) -> ()  [unwired: 8 in, 2 out]
          }
          frame "Commands" {
            w385 = u32 5789784 ("Color Box")
            w386 = T27 {"Row"=-1, "Column"=-2} ("Active Cell:Active Cell")
            w388 = T27 {"Row"=-2, "Column"=-2} ("Active Cell:Active Cell")
            n220 = Index Array(array=w389, index=w383) -> (element=w387:u32)
            n221 = Index Array(array=w384, index=w383) -> (element=w382:T26)
            n222 = Unbundle(w382) -> ("Operation"=w381:enum16{"Update", "Clear"})  [unwired: 1 out]
            n223 = local read "Command Selection"() -> (w380:i32)
            n224 = property on="Command Selection" class="MCListbox (strict)"("ActiveCell"=w388, "CellBG"=w387, "ActiveCell"=w386, "CellBG"=w385) -> ()  [unwired: 2 in, 2 out]
            n225 = call <vilib>:"WPI_DashboardUpdate RPC Info.vi"("Operation"=w381) -> ("update"=w379:bool, "commands"=w378:string[][])  [unwired: 9 in]
            n226 = property on="Command Selection" class="MCListbox (strict)"("ItemNames"=w378) -> ()  [unwired: 2 in, 2 out]
            n227 = property on="Command Params" class="Tbl (strict)"("Active Cell"=w388, "Cell BG Color"=w387, "Active Cell"=w386, "Cell BG Color"=w385) -> ()  [unwired: 2 in, 2 out]
            n228 = call <vilib>:"WPI_DashboardUpdate Command Params.vi"("Update"=w379, "NewVal"=w380, "Commands"=w378, "Param Tbl"=w377) -> ()  [unwired: 7 in, 1 out]
          }
        }
        n229 = call <vilib>:"Connextion Info.vi"() -> ("Connected"=→"NT Connection":bool)  [unwired: 10 in, 1 out]
      }
      event "Test Tree": Value Change {
        # "Show appropriate\ncontrols"
        n230 = event-data() -> ("CtlRef"=w394:refnum<vi>, "NewVal"=w392:string)  [unwired: 1 in]
        n231 = call <vilib>:"WPI_UtilitiesGetTreeIOName.vi"("NewVal"=w392, "TreeControl in"=w394) -> ("I/O Name"=w395:string)  [unwired: 9 in]
        n232 = case shown="\"Camera\"" w395 {
          selector: w395 -> [_ w402 _ w424 w433 _]
          tunnel: w392 -> [_ _ w421 w423 _ w440]
          tunnel: cluster{string[]}[] [{["640x480", "320x240", "160x120"]}, {["Auto", "Fixed indoor", "Fixed outdoor 1", "Fixed outdoor 2", "Fixed fluorescent 1", "Fixed fluorescent 2", "Hold current"]}, {["Auto", "Flicker-free 50 Hz", "Flicker-free 60 Hz", "Hold current"]}, {["None", "Prioritize frame rate", "Prioritize image quality"]}, {["Monochrome", "Color"]}] -> [_ _ _ _ _ w439]
          frame Default {
            w397 = FALSE ("Visible")
            w396 = FALSE ("Visible")
            n233 = property on="Motor" class="Clust (strict)"("Visible"=w396) -> ()  [unwired: 2 in, 2 out]
            n234 = property on="Test Ring" class="Ring (strict)"("Visible"=w396) -> ()  [unwired: 2 in, 2 out]
            n235 = property on="Rev/Fwd" class="Clust (strict)"("Visible"=w397) -> ()  [unwired: 2 in, 2 out]
            n236 = property on="On/Off" class="Bool (strict)"("Visible"=w397) -> ()  [unwired: 2 in, 2 out]
            n237 = property on="Test Slider" class="Slide (strict)"("Visible"=w397) -> ()  [unwired: 2 in, 2 out]
          }
          frame "Analog Out", "Motor", "PWM" {
            w403 = FALSE ("Visible")
            n238 = case shown="\"Analog Out\"" w402 {
              tunnel: [1.0 ("Value") -1.0 ("Value") 0.0 ("Value")] -> w401
              tunnel: [255.0 ("Value") 1.0 ("Value") 5.0 ("Value")] -> w400
              tunnel: [128.0 ("Value") 0.0 ("Value") 0.0 ("Value")] -> w399
              tunnel: [64.0 ("Value") 0.5 ("Value") 1.0 ("Value")] -> w398
              frame "PWM" {
              }
              frame "Motor", Default {
              }
              frame "Analog Out" {
              }
            }
            n239 = property on="Motor" class="Clust (strict)"("Visible"=TRUE) -> ()  [unwired: 2 in, 2 out]
            n240 = property on="Value" class="Slide (strict)"("Value"=w399, "Scale.Minimum"=w401, "Scale.Maximum"=w400, "Scale.Increment"=w398) -> ()  [unwired: 2 in, 2 out]
            n241 = property on="On/Off" class="Bool (strict)"("Visible"=w403) -> ()  [unwired: 2 in, 2 out]
            n242 = property on="Test Slider" class="Slide (strict)"("Visible"=w403) -> ()  [unwired: 2 in, 2 out]
            n243 = property on="Test Ring" class="Ring (strict)"("Visible"=w403) -> ()  [unwired: 2 in, 2 out]
            n244 = property on="Rev/Fwd" class="Clust (strict)"("Visible"=w403) -> ()  [unwired: 2 in, 2 out]
          }
          frame "Servo" {
            w419 = FALSE ("Visible")
            n245 = call <vilib>:"NT Read Number.vi"("Name"=w421) -> ("Numeric"=w420:dbl)  [unwired: 9 in, 1 out]
            n246 = property on="Test Slider" class="Slide (strict)"("Visible"=TRUE, "Scale.Maximum"=170.0 ("Scale.Range:Maximum")) -> ()  [unwired: 2 in, 2 out]
            n247 = local write "Test Slider"(w420) -> ()
            n248 = property on="Motor" class="Clust (strict)"("Visible"=w419) -> ()  [unwired: 2 in, 2 out]
            n249 = property on="Rev/Fwd" class="Clust (strict)"("Visible"=w419) -> ()  [unwired: 2 in, 2 out]
            n250 = property on="On/Off" class="Bool (strict)"("Visible"=w419) -> ()  [unwired: 2 in, 2 out]
            n251 = property on="Test Ring" class="Ring (strict)"("Visible"=w419) -> ()  [unwired: 2 in, 2 out]
          }
          frame "Relay", "Solenoid" {
            w422 = FALSE ("Visible")
            n252 = property on="Motor" class="Clust (strict)"("Visible"=w422) -> ()  [unwired: 2 in, 2 out]
            n253 = property on="Test Slider" class="Slide (strict)"("Visible"=w422) -> ()  [unwired: 2 in, 2 out]
            n254 = Search and Replace String(input string=w423, search string="/Value  **", replace string="/Direction") -> (result string=w429:string)  [unwired: 5 in, 3 out]
            n255 = property on="Test Ring" class="Ring (strict)"("Visible"=w422) -> ()  [unwired: 2 in, 2 out]
            n256 = call <vilib>:"NT Read String.vi"("Name"=w429) -> ("String"=w427:string)  [unwired: 9 in, 1 out]
            n257 = Equal?(x="Both directions", y=w427) -> (x = y?=w425:bool)
            n258 = Not(x=w425) -> (.not. x?=w426:bool)
            n259 = property on="Rev/Fwd" class="Clust (strict)"("Visible"=w425) -> ()  [unwired: 2 in, 2 out]
            n260 = property on="On/Off" class="Bool (strict)"("Visible"=w426, "Caption.Text"=w424) -> ()  [unwired: 2 in, 2 out]
          }
          frame "Compressor", "Digital Out" {
            w432 = FALSE ("Visible")
            # "Get direction and finish"
            n261 = property on="Motor" class="Clust (strict)"("Visible"=w432) -> ()  [unwired: 2 in, 2 out]
            n262 = property on="Test Slider" class="Slide (strict)"("Visible"=w432) -> ()  [unwired: 2 in, 2 out]
            n263 = property on="Test Ring" class="Ring (strict)"("Visible"=w432) -> ()  [unwired: 2 in, 2 out]
            n264 = property on="On/Off" class="Bool (strict)"("Visible"=TRUE, "Caption.Text"=w433) -> ()  [unwired: 2 in, 2 out]
            n265 = property on="Rev/Fwd" class="Clust (strict)"("Visible"=FALSE) -> ()  [unwired: 2 in, 2 out]
          }
          frame "Camera" {
            n266 = call <vilib>:"Get Last Path Segment.vi"("String in"=w440) -> ("String out"=w441:string)  [unwired: 10 in]
            n267 = property on="On/Off" class="Bool (strict)"("Visible"=FALSE) -> ()  [unwired: 2 in, 2 out]
            n268 = property on="Motor" class="Clust (strict)"("Visible"=FALSE) -> ()  [unwired: 2 in, 2 out]
            n269 = property on="Rev/Fwd" class="Clust (strict)"("Visible"=FALSE) -> ()  [unwired: 2 in, 2 out]
            n270 = case shown="\"White Balance  **\"" w441 {
              tunnel: w440 -> [w447 w456 w465 w474 w483 _ w489]
              tunnel: w439 -> [w445 w453 w462 w471 w480 _ _]
              frame "Size  **" {
                n271 = Index Array(array=w445) -> (element=w444:cluster{string[]})  [unwired: 1 in]
                n272 = call <vilib>:"NT Read String.vi"("Name"=w447) -> ("String"=w446:string)  [unwired: 9 in, 1 out]
                n273 = Unbundle(w444) -> (w442:string[])
                n274 = Match First String(2:w442, 3:w446) -> (0:w443:i32)  [unwired: 1 out]
                n275 = property on="Test Ring" class="Ring (strict)"("Value"=w443, "Strings []"=w442) -> ()  [unwired: 2 in, 2 out]
                n276 = property on="Test Ring" class="Ring (strict)"("Visible"=TRUE) -> ()  [unwired: 2 in, 2 out]
                n277 = property on="Test Slider" class="Slide (strict)"("Visible"=FALSE) -> ()  [unwired: 2 in, 2 out]
              }
              frame "White Balance  **" {
                n278 = Index Array(array=w453, index=1) -> (element=w454:cluster{string[]})
                n279 = call <vilib>:"NT Read String.vi"("Name"=w456) -> ("String"=w455:string)  [unwired: 9 in, 1 out]
                n280 = Unbundle(w454) -> (w451:string[])
                n281 = Match First String(2:w451, 3:w455) -> (0:w450:i32)  [unwired: 1 out]
                n282 = property on="Test Ring" class="Ring (strict)"("Value"=w450, "Strings []"=w451) -> ()  [unwired: 2 in, 2 out]
                n283 = property on="Test Ring" class="Ring (strict)"("Visible"=TRUE) -> ()  [unwired: 2 in, 2 out]
                n284 = property on="Test Slider" class="Slide (strict)"("Visible"=FALSE) -> ()  [unwired: 2 in, 2 out]
              }
              frame "Exposure  **" {
                n285 = Index Array(array=w462, index=2) -> (element=w463:cluster{string[]})
                n286 = call <vilib>:"NT Read String.vi"("Name"=w465) -> ("String"=w464:string)  [unwired: 9 in, 1 out]
                n287 = Unbundle(w463) -> (w459:string[])
                n288 = Match First String(2:w459, 3:w464) -> (0:w460:i32)  [unwired: 1 out]
                n289 = property on="Test Ring" class="Ring (strict)"("Value"=w460, "Strings []"=w459) -> ()  [unwired: 2 in, 2 out]
                n290 = property on="Test Ring" class="Ring (strict)"("Visible"=TRUE) -> ()  [unwired: 2 in, 2 out]
                n291 = property on="Test Slider" class="Slide (strict)"("Visible"=FALSE) -> ()  [unwired: 2 in, 2 out]
              }
              frame "Exposure Priority  **" {
                n292 = Index Array(array=w471, index=3) -> (element=w472:cluster{string[]})
                n293 = call <vilib>:"NT Read String.vi"("Name"=w474) -> ("String"=w473:string)  [unwired: 9 in, 1 out]
                n294 = Unbundle(w472) -> (w468:string[])
                n295 = Match First String(2:w468, 3:w473) -> (0:w469:i32)  [unwired: 1 out]
                n296 = property on="Test Ring" class="Ring (strict)"("Value"=w469, "Strings []"=w468) -> ()  [unwired: 2 in, 2 out]
                n297 = property on="Test Ring" class="Ring (strict)"("Visible"=TRUE) -> ()  [unwired: 2 in, 2 out]
                n298 = property on="Test Slider" class="Slide (strict)"("Visible"=FALSE) -> ()  [unwired: 2 in, 2 out]
              }
              frame "Color Enable  **" {
                n299 = Index Array(array=w480, index=4) -> (element=w481:cluster{string[]})
                n300 = call <vilib>:"NT Read String.vi"("Name"=w483) -> ("String"=w482:string)  [unwired: 9 in, 1 out]
                n301 = Unbundle(w481) -> (w477:string[])
                n302 = Match First String(2:w477, 3:w482) -> (0:w478:i32)  [unwired: 1 out]
                n303 = property on="Test Ring" class="Ring (strict)"("Value"=w478, "Strings []"=w477) -> ()  [unwired: 2 in, 2 out]
                n304 = property on="Test Ring" class="Ring (strict)"("Visible"=TRUE) -> ()  [unwired: 2 in, 2 out]
                n305 = property on="Test Slider" class="Slide (strict)"("Visible"=FALSE) -> ()  [unwired: 2 in, 2 out]
              }
              frame Default {
                n306 = property on="Test Ring" class="Ring (strict)"("Visible"=FALSE) -> ()  [unwired: 2 in, 2 out]
                n307 = property on="Test Slider" class="Slide (strict)"("Visible"=FALSE) -> ()  [unwired: 2 in, 2 out]
              }
              frame "Brightness  **", "Color Level  **", "Compression  **", "FPS  **", "Sharpness  **" {
                n308 = call <vilib>:"NT Read Number.vi"("Name"=w489) -> ("Numeric"=w488:dbl)  [unwired: 9 in, 1 out]
                n309 = local write "Test Slider"(w488) -> ()
                n310 = property on="Test Slider" class="Slide (strict)"("Visible"=TRUE, "Scale.Maximum"=100.0 ("Scale.Range:Maximum")) -> ()  [unwired: 2 in, 2 out]
                n311 = property on="Test Ring" class="Ring (strict)"("Visible"=FALSE) -> ()  [unwired: 2 in, 2 out]
              }
            }
          }
        }
        n312 = property on="Progress" class="Clust (strict)"("Visible"=FALSE) -> ()  [unwired: 2 in, 2 out]
      }
      event "Test Name": Mouse Enter {
        # "Populate the ring with the list of tests"
        n313 = event-data() -> ()  [unwired: 1 in, 1 out]
        n314 = call <vilib>:"NT Read String Array.vi"("Name"="TestMode/TestList") -> ("String Array"=w497:string[])  [unwired: 9 in, 1 out]
        n315 = Build Array (concatenate)("Select the test to run...", w497) -> (w496:string[])
        n316 = property on="Test Name" class="Ring (strict)"("Strings []"=w496) -> ()  [unwired: 2 in, 2 out]
      }
      event "Test Name": Value Change {
        w499 = FALSE ("Visible")
        # "Tell the robot the test name to run"
        n317 = event-data() -> ("NewVal"=w503:u16)  [unwired: 1 in]
        n318 = property on="Test Name" class="Ring (strict)"() -> ("Strings []"=w504:string[])  [unwired: 2 in, 2 out]
        n319 = local write "Progress"(T6 {"Test Progress"=0, "Test Progress Text"=""} ("Progress")) -> ()
        n320 = Index Array(array=w504, index=w503) -> (element=w502:string)
        n321 = call <vilib>:"NT Write String.vi"("String"=w502, "Name"="TestMode/TestName") -> ()  [unwired: 9 in, 1 out]
        n322 = property on="Progress" class="Clust (strict)"("Visible"=TRUE) -> ()  [unwired: 2 in, 2 out]
        n323 = property on="Motor" class="Clust (strict)"("Visible"=w499) -> ()  [unwired: 2 in, 2 out]
        n324 = property on="Test Slider" class="Slide (strict)"("Visible"=w499) -> ()  [unwired: 2 in, 2 out]
        n325 = property on="On/Off" class="Bool (strict)"("Visible"=w499) -> ()  [unwired: 2 in, 2 out]
        n326 = property on="Rev/Fwd" class="Clust (strict)"("Visible"=w499) -> ()  [unwired: 2 in, 2 out]
        n327 = property on="Test Ring" class="Ring (strict)"("Visible"=w499) -> ()  [unwired: 2 in, 2 out]
      }
      event "Select Auto": Mouse Enter {
        # "Populate the combo box with the list of autonomous options"
        n328 = event-data() -> ()  [unwired: 1 in, 1 out]
        n329 = call <vilib>:"NT Read String Array.vi"("Name"="Auto List") -> ("String Array"=w506:string[])  [unwired: 9 in, 1 out]
        n330 = property on="Select Auto" class="CmbBox"("Strings[]"=w506) -> ()  [unwired: 2 in, 2 out]
      }
      event "Select Auto": Value Change {
        # "User modified the Auto Selection. Write to NT variable so robot knows."
        n331 = event-data() -> ("NewVal"=w509:string)  [unwired: 1 in]
        n332 = call <vilib>:"NT Write String.vi"("String"=w509, "Name"="Auto Selector") -> ()  [unwired: 9 in, 1 out]
      }
      event "Command Selection": Value Change {
        # "Get the params and show in table"
        n333 = event-data() -> ("NewVal"=w515:i32)  [unwired: 1 in]
        n334 = property on="Command Selection" class="MCListbox (strict)"() -> ("ItemNames"=w513:string[][])  [unwired: 2 in, 2 out]
        n335 = call <vilib>:"WPI_DashboardUpdate Command Params.vi"("NewVal"=w515, "Commands"=w513, "Param Tbl"=w514) -> ()  [unwired: 8 in, 1 out]
      }
      event "Execute Command": Value Change {
        # "Started one, Unique ID holds\nresponse"
        n336 = event-data() -> ()  [unwired: 1 in, 1 out]
        n337 = property on="Command Selection" class="MCListbox (strict)"() -> ("ItemNames"=w526:string[][])  [unwired: 2 in, 2 out]
        n338 = Index Array(array=w526, index (row)="Command Selection", index (col)=0) -> (element=w524:string)
        n339 = call <vilib>:"Invoke Commands.vi"("Command Params"="Command Params", "Function Name"=w524) -> ("Params"=w520:u8, "Started"=w519:bool)  [unwired: 7 in, 1 out]
        n340 = Array Subset(array="Command Params", length (row)=w520) -> (w521:string[][])  [unwired: 3 in]
        n341 = Select(t="Executing" ("Cmd Status"), s=w519, f="" ("Cmd Status")) -> (s? t:f=→"Cmd Status":string)
      }
      event "Command Selection": Double Click {
        n342 = event-data() -> ("Row"=w534:i32)  [unwired: 1 in]
        n343 = property on="Command Selection" class="MCListbox (strict)"() -> ("ItemNames"=w537:string[][])  [unwired: 2 in, 2 out]
        n344 = local read "Command Params"() -> (w533:string[][])
        n345 = Index Array(array=w537, index (row)=w534, index (col)=0) -> (element=w535:string)
        n346 = call <vilib>:"Invoke Commands.vi"("Command Params"=w533, "Function Name"=w535) -> ("Params"=w532:u8, "Started"=w527:bool)  [unwired: 7 in, 1 out]
        n347 = Array Subset(array=w533, length (row)=w532) -> (w531:string[][])  [unwired: 3 in]
        n348 = Select(t="Executing" ("Cmd Status"), s=w527, f="" ("Cmd Status")) -> (s? t:f=w528:string)
        n349 = local write "Cmd Status"(w528) -> ()
      }
      event "CheckList": Double Click {
        # "Shift clears all"
        # "Update symbols on the listbox"
        n350 = event-data() -> ("PlatMods.Shift"=w539:bool, "Row"=w541:i32)  [unwired: 1 in]
        n351 = case shown="True" w539 {
          tunnel: w541 -> [w545 _]
          tunnel: 1 -> [w544 _]
          frame False {
            n352 = property on="CheckList" class="LstBox (strict)"() -> ("Item Symbols"=w543:i32[])  [unwired: 2 in, 2 out]
            n353 = Replace Array Subset(array=w543, new element=w544, index=w545) -> (w542:i32[])
            n354 = property on="CheckList" class="LstBox (strict)"("Item Symbols"=w542) -> ()  [unwired: 2 in, 2 out]
          }
          frame True {
            w546 = 0 ("Top Row")
            n355 = property on="CheckList" class="LstBox (strict)"() -> ("Number of Rows"=w548:u32)  [unwired: 2 in, 2 out]
            n356 = Initialize Array(0, w548) -> (w547:i32[])
            n357 = property on="CheckList" class="LstBox (strict)"("Top Row"=w546, "Value"=w546, "Item Symbols"=w547) -> ()  [unwired: 2 in, 2 out]
          }
        }
      }
      event "CheckList": Key Down {
        # "Update symbols on the listbox\nLeft and right keys check and uncheck"
        n358 = event-data() -> ("VKey"=w552:T24)  [unwired: 1 in]
        n359 = case shown="\"Left\", \"Right\"" w552 {
          selector: w552 -> [w557 _]
          tunnel: eventvkey."Left" ("VKey") -> [w555 _]
          frame "Left", "Right" {
            n360 = Equal?(x=w555, y=w557) -> (x = y?=w556:bool)
            n361 = Select(t=0, s=w556, f=1) -> (s? t:f=w558:i32)
            n362 = property on="CheckList" class="LstBox (strict)"() -> ("Item Symbols"=w561:i32[])  [unwired: 2 in, 2 out]
            n363 = Replace Array Subset(array=w561, new element=w558, index="CheckList") -> (w560:i32[])
            n364 = property on="CheckList" class="LstBox (strict)"("Item Symbols"=w560) -> ()  [unwired: 2 in, 2 out]
          }
          frame Default {
          }
        }
      }
      event "Motor.Enable": Value Change {
        # "When the test mode otor enable helper is set, update that\ntree row item's value"
        n365 = event-data() -> ("NewVal"=w567:bool)  [unwired: 1 in]
        n366 = Unbundle("Motor") -> ("Value"=w566:dbl)  [unwired: 1 out]
        n367 = Select(t=w566, s=w567, f=0.0) -> (s? t:f=w564:dbl)
        n368 = call <vilib>:"NT Write Number.vi"("Numeric"=w564, "Name"=w563) -> ()  [unwired: 9 in, 1 out]
      }
      event "Test Slider": Value Change {
        # "When the test mode slider helper is set, update that\ntree row item's value"
        n369 = event-data() -> ("NewVal"=w570:dbl)  [unwired: 1 in]
        n370 = call <vilib>:"NT Write Number.vi"("Numeric"=w570, "Name"=w571) -> ()  [unwired: 9 in, 1 out]
      }
      event "On/Off": Value Change {
        # "When the test mode on/off helper value is set, update that\ntree row item's value"
        n371 = event-data() -> ("NewVal"=w575:bool)  [unwired: 1 in]
        n372 = Boolean To (0,1)(Boolean=w575) -> (0, 1=w574:i16)
        n373 = call <vilib>:"NT Write Number.vi"("Numeric"=w574, "Name"=w573) -> ()  [unwired: 9 in, 1 out]
      }
      event "Rev/Fwd": Value Change {
        # "When the test mode helper value for relays is set, update that\ntree row item's value"
        n374 = event-data() -> ("NewVal.Forward"=w583:bool, "NewVal.Reverse"=w582:bool)  [unwired: 1 in]
        n375 = Boolean To (0,1)(Boolean=w583) -> (0, 1=w579:i16)
        n376 = Boolean To (0,1)(Boolean=w582) -> (0, 1=w581:i16)
        n377 = Negate(x=w581) -> (-x=w580:i16)
        n378 = Add(x=w579, y=w580) -> (x+y=w578:i16)
        n379 = call <vilib>:"NT Write Number.vi"("Numeric"=w578, "Name"=w577) -> ()  [unwired: 9 in, 1 out]
      }
      event "Test Ring": Value Change {
        # "When a test mode helper value is selected from the ring,\nset the tree item's variable to the string value"
        n380 = event-data() -> ("NewVal"=w587:u16)  [unwired: 1 in]
        n381 = property on="Test Ring" class="Ring (strict)"() -> ("Strings []"=w588:string[])  [unwired: 2 in, 2 out]
        n382 = Index Array(array=w588, index=w587) -> (element=w586:string)
        n383 = call <vilib>:"NT Write String.vi"("String"=w586, "Name"=w585) -> ()  [unwired: 9 in, 1 out]
      }
      event "Rec Mode": Value Change {
        # "Update globals for recording mode and path to read log from.\nClear when logging and let NetworkTables set path for vision to\nuse."
        n384 = event-data() -> ("NewVal"=w599:enum32{"Stop", "Record", "Playback"})  [unwired: 1 in]
        n385 = global write "WPI_DashboardLogging Global.vi" "Logging Filename"(path "") -> ()
        n386 = global write "WPI_DashboardLogging Global.vi" "Recording"(w599) -> ()
        n387 = case shown="\"Playback\"" w599 {
          tunnel: w598 -> [_ w601 w610]
          tunnel: [_ _ w609] -> w596
          tunnel: [_ _ w608] -> _
          tunnel: w594 -> [_ _ w606]
          tunnel: cluster{i32, i32} {-250, 170} -> [_ _ w605]
          tunnel: [_ _ T25 {"Image Size"=TRUE, "Image Type"=TRUE, "Pixel Value"=TRUE, "ROI Information"=TRUE, "Zoom Factor"=FALSE} ("Image Information Shown:All Elements")] -> w589
          tunnel: [_ _ TRUE ("Zoom Factor")] -> w590
          tunnel: w592 -> [_ _ w602]
          frame Default {
          }
          frame "Stop", "Record" {
            # "Place Window too"
            n388 = invoke class="VI" method="FP.Close"(reference=w601) -> (reference out=w600:refnum<vi>)  [unwired: 2 in, 2 out]
            n389 = invoke class="VI" method="Abort VI"(reference=w600) -> ()  [unwired: 2 in, 3 out]
          }
          frame "Playback" {
            n390 = call "Open Playback Panel.vi"("Offset"=w605, "DB VI Ref"=w606, "Playback in"=w610) -> ("Playback out"=w607:refnum<vi>)  [unwired: 8 in]
            n391 = register-events(w607, w602) -> (reference out=w609:refnum<event-registration>, error out=w608:errorcluster)  [unwired: 2 in]
          }
        }
        n392 = property on="Camera Image Right" class="ImageControl"("Image Information Shown"=w589, "Image Information Visible"=w590) -> ()  [unwired: 2 in, 2 out]
        n393 = property on="Camera Image" class="ImageControl"("Image Information Shown"=w589, "Image Information Visible"=w590) -> ()  [unwired: 2 in, 2 out]
        n394 = call <vilib>:"WPI_DashboardNT Log FieldName Cache.vi"("Operation"=enum16{"Lookup/Add", "Index", "Clear"}."Clear") -> ()  [unwired: 8 in, 3 out]
      }
      event Panel Close {
        w612 = enum32{"Stop", "Record", "Playback"}."Stop" ("Rec Mode")
        # "Playback window has been closed, abort"
        n395 = event-data() -> ()  [unwired: 1 in, 4 out]
        n396 = local write "Rec Mode"(w612) -> ()
        n397 = global write "WPI_DashboardLogging Global.vi" "Recording"(w612) -> ()
      }
      event Panel Close {
        # "Abort playback window and ourself"
        n398 = event-data() -> ()  [unwired: 1 in, 4 out]
        n399 = invoke class="VI" method="FP.Close"(reference=w616) -> (reference out=w615:refnum<vi>)  [unwired: 2 in, 2 out]
        n400 = invoke class="VI" method="Abort VI"(reference=w615) -> (error out=w614:errorcluster)  [unwired: 2 in, 2 out]
        n401 = invoke class="VI" method="Abort VI"(error in=w614) -> ()  [unwired: 2 in, 3 out]
      }
      event User Event {
        n402 = event-data() -> ("IDs"=w623:cluster{"RPC field ID":u16, "Unique ID":u16}, "String"=w622:string)  [unwired: 1 in]
        n403 = Bundle("IDs"=w623, "String"=w622) -> (w621:T11)  [unwired: 1 in]
        n404 = call <vilib>:"Retrieve RPC Response.vi"("RPC Response"=w621) -> ("Output"=w619:string[][])  [unwired: 10 in]
        n405 = Build Array (concatenate)(w617, w619) -> (w618:string[][])
        n406 = local write "Command Params"(w618) -> ()
        n407 = local write "Cmd Status"("" ("Cmd Status")) -> ()
      }
      event "Tree": Double Click {
        n408 = event-data() -> ("PlatMods"=w629:T28, "Tag"=w626:string)  [unwired: 1 in]
        n409 = Unbundle(w629) -> ("Shift"=w628:bool)  [unwired: 4 out]
        n410 = String Subset(string=w626, length (rest)=1 ("length (rest)")) -> (substring=w625:string)  [unwired: 1 in]
        n411 = Not(x=w628) -> (.not. x?=w627:bool)
        n412 = case shown="\"/\"" w625 {
          tunnel: w626 -> [_ w632]
          tunnel: w627 -> [_ w631]
          frame Default {
          }
          frame "/" {
            n413 = call <vilib>:"NT Update Persistence.vi"("Persistence"=w631, "Name"=w632) -> ()  [unwired: 9 in, 1 out]
          }
        }
      }
    }
  }
  n414 = while {
    tunnel: w80 -> [w634]
    i -> [w637]
    stop <- FALSE stop-if-true
    n415 = Wait (ms)(milliseconds to wait=u32 100) -> ()  [unwired: 1 out]
    n416 = case shown="\"Playback\"" "Rec Mode" {
      tunnel: w637 -> [_ _ w652]
      tunnel: [u32 2829099 ("Base Color") u32 11141120 ("Target Color") w641] -> w633
      frame "Stop", Default {
        # "Reset the color, extra updates don't cost much"
      }
      frame "Record" {
      }
      frame "Playback" {
        # "Playback"
        n417 = Quotient & Remainder(x=w652, y=u32 50 ("milliseconds to wait")) -> (x-y*floor(x/y)=w648:u32)  [unwired: 1 out]
        n418 = Divide(x=w648, y=u32 50 ("milliseconds to wait")) -> (x/y=w645:dbl)
        n419 = Multiply(x=6.283185307179586, y=w645) -> (x*y=w650:dbl)
        n420 = Sine(x=w650) -> (sin(x)=w649:dbl)
        n421 = Absolute Value(x=w649) -> (abs(x)=w642:dbl)
        n422 = call "Interpolate RGB Color.vi"("Proportion"=w642, "Target Color"=u32 30976, "Base Color"=u32 2829099) -> ("Result Color"=w641:u32)  [unwired: 8 in]
      }
    }
    n423 = property class="Pane"(reference=w634, "PaneColor"=w633) -> ()  [unwired: 1 in, 2 out]
  }
  n424 = local write "Dashboard Tab"(T9."Drive" ("Dashboard Tab")) -> ()
  n425 = property on="On/Off" class="Bool (strict)"("Visible"=w51) -> ()  [unwired: 2 in, 2 out]
  n426 = property on="Motor" class="Clust (strict)"("Visible"=w51) -> ()  [unwired: 2 in, 2 out]
  n427 = property on="Progress" class="Clust (strict)"("Visible"=w51) -> ()  [unwired: 2 in, 2 out]
  n428 = property on="Test Ring" class="Ring (strict)"("Visible"=w51) -> ()  [unwired: 2 in, 2 out]
  n429 = property on="Rev/Fwd" class="Clust (strict)"("Visible"=w51) -> ()  [unwired: 2 in, 2 out]
  n430 = while {
    tunnel: u16 1741 ("timeout ms (25000)") -> [w654]
    stop <- FALSE stop-if-true
    n431 = TCP Create Listener(10:w654) -> (0:w653:errorcluster, 3:w655:refnum<k5>)  [unwired: 4 in, 1 out]
    n432 = case shown="Error" w653 {
      selector: w653 -> [w657 _]
      tunnel: w655 -> [w658 _]
      frame No Error {
        n433 = while {
          tunnel: w658 -> [w661]
          tunnel: w657 -> [w660]
          stop <- FALSE stop-if-true
          n434 = TCP Wait On Listener(8:w660, 11:w661) -> (0:w662:errorcluster, 4:w663:refnum<k5>)  [unwired: 2 in, 3 out]
          n435 = local write "TCP"(w663) -> ()
          n436 = case shown="No Error" w662 {
            frame No Error {
            }
            frame Error {
              n437 = Wait (ms)(milliseconds to wait=u32 1000) -> ()  [unwired: 1 out]
            }
          }
        }
      }
      frame Error {
        n438 = Wait (ms)(milliseconds to wait=u32 1000) -> ()  [unwired: 1 out]
      }
    }
  }
  n439 = local write "Command Selection"(u16 0 ("milliseconds to wait")) -> ()
  n440 = local write "Command Params"(string[][] [] ("Command Params")) -> ()
  n441 = global write "WPI_DashboardLogging Global.vi" "Recording"(w74) -> ()
  n442 = local write "Rec Mode"(w74) -> ()
  n443 = call <vilib>:"NT Write String.vi"("String"="Select Auto", "Name"="Auto Selector") -> ()  [unwired: 9 in, 1 out]
